vi "MainController4.vi"() -> ()   [LabVIEW 2009]
doc: "The top-level VI for the SRV application.\n\n\nModified: Mike Schultz - Logic PD"
uses:
  SRV VIs/ImageProcessing/QT_Image.ctl
  SRV VIs/SubVIs/SRV_Response Data Type.ctl
  SRV VIs/Motors/Motors Config/SRV_Motor Control Button Icons_TRUE.ctl
  SRV VIs/Motors/Motors Config/SRV_Motor Control Button Icons_FALSE.ctl
  SRV VIs/SubVIs/SRV_SRV_Loops Notifier Methods.ctl
  SRV VIs/SRV_Main Controller Local Data.ctl
  SRV VIs/Motors/Motors Config/SRV_Motor Control Button Config.ctl
  SRV VIs/Motors/Motors Config/SRV_Motor Legos-Servo.ctl
  SRV VIs/Motors/Motors Config/SRV_Motor Control Commands Cluster.ctl
  SRV VIs/Motors/Motors Config/SRV_Motor Control Command Config.ctl
  SRV VIs/SubVIs/SRV_Streaming States.ctl
  SRV VIs/SubVIs/SRV_Streaming State.ctl
  SRV VIs/PacketMode/SRV_PM_Packet.ctl
  SRV VIs/Support/SRV_Command-Data Queue Data Type.ctl
  SRV VIs/PacketMode/SRV_PM_Packet Mode Style.ctl
  SRV VIs/Motors/SRV_Button Event Data.ctl
  SRV VIs/SubVIs/SRV_Streaming Modes.ctl
  <vilib>/Utility/miscctls.llb/LVBoundsTypeDef.ctl
  SRV VIs/SubVIs/SRV_Number of IMJ Requests Methods.ctl
  SRV VIs/SubVIs/SRVGlobals.vi
panel:
  in  "button E5":bool
  out "true E5":T1
  out "false E5":T2
  in  "button E4":bool
  out "true E4":T1
  out "false E4":T2
  in  "button E3":bool
  out "true E3":T1
  out "false E3":T2
  in  "button E1":bool
  out "true E1":T1
  out "false E1":T2
  in  "button E2":bool
  out "true E2":T1
  out "false E2":T2
  in  "button E7":bool
  out "true E7":T1
  out "false E7":T2
  in  "button E6":bool
  out "true E6":T1
  out "false E6":T2
  in  "button D7":bool
  out "true D7":T1
  out "false D7":T2
  in  "button A7":bool
  out "true A7":T1
  out "false A7":T2
  in  "button C7":bool
  out "true C7":T1
  out "false C7":T2
  in  "button B7":bool
  out "true B7":T1
  out "false B7":T2
  in  "button D6":bool
  out "true D6":T1
  out "false D6":T2
  in  "button A6":bool
  out "true A6":T1
  out "false A6":T2
  in  "button C6":bool
  out "true C6":T1
  out "false C6":T2
  in  "button B6":bool
  out "true B6":T1
  out "false B6":T2
  in  "button D5":bool
  out "true D5":T1
  out "false D5":T2
  in  "button A5":bool
  out "true A5":T1
  out "false A5":T2
  in  "button C5":bool
  out "true C5":T1
  out "false C5":T2
  in  "button B5":bool
  out "true B5":T1
  out "false B5":T2
  in  "button D4":bool
  out "true D4":T1
  out "false D4":T2
  in  "button A4":bool
  out "true A4":T1
  out "false A4":T2
  in  "button C4":bool
  out "true C4":T1
  out "false C4":T2
  in  "button B4":bool
  out "true B4":T1
  out "false B4":T2
  in  "button D3":bool
  out "true D3":T1
  out "false D3":T2
  in  "button A3":bool
  out "true A3":T1
  out "false A3":T2
  in  "button C3":bool
  out "true C3":T1
  out "false C3":T2
  in  "button B3":bool
  out "true B3":T1
  out "false B3":T2
  in  "button D2":bool
  out "true D2":T1
  out "false D2":T2
  in  "button A2":bool
  out "true A2":T1
  out "false A2":T2
  in  "button C2":bool
  out "true C2":T1
  out "false C2":T2
  in  "button B2":bool
  out "true B2":T1
  out "false B2":T2
  in  "Expand-Collapse":bool
  in  "button D1":bool
  out "true D1":T1
  out "false D1":T2
  in  "button A1":bool
  out "true A1":T1
  out "false A1":T2
  in  "button C1":bool
  out "true C1":T1
  out "false C1":T2
  in  "button B1":bool
  out "true B1":T1
  out "false B1":T2
  out "Overflow Indicator":bool
  out "ms Diff 3":u32
  out "ms Diff 2":u32
  out "ms Diff parse":u32
  out "ms Diff ##IMJ":u32
  out "ms Diff DQ":u32
  out "ms Diff":u32
  out "Response Data Type":T3=enum."No Data"
  out "i4":i32
  in  "Show Image":bool
  out "InPico State Change":bool
  in  "clear":bool
  out "Replies":string
  out "Number of IMJ Requests":i32
  out "XModem Replies":string[](array[string])
  out "i1":i32
  out "i2":i32
  out "Status":string
  out "The image":picture caption="new picture"
  out "SRV Out":refnum<k5>
  out "SRV IP Address":string
  out "In Pico":bool
  out "connected?":bool
  in  "Tab Control":T4(tab)
  in  "Send Text":bool
  in  "ESC":bool
  in  "Direct Command to Send":string
  in  "Run CCode":bool
  in  "View Code":bool
  in  "Upload CCode":bool
  in  "C Code":string="int x,y,z;\nfor (x = 0; x < 2; x++) \n  {  \n    for (y = 0; y < 3; y++)\n       {       \n         for (z = 0; z < 2; z++)\n           {\n             printf(\"%d %d %d\\n\", x,y,z);   \n           }\n        } \n   }\nexit(1);"
  in  "load Text":bool
  out "Cover":bool
  out "Last file name":string
  in  "Movie Mode":bool
  in  "Path to folder":path
  in  "Snap":bool
  out "YUV_SRV":cluster{"Y":sgl, "U":sgl, "V":sgl}
  in  "Threshold":i8(slide)=4 scale=1.0..9.0
  in  "Plan":T5(radio)
  in  "Bins":T6(ring)=enum."4 levels of U and 4 levels of V"
  out "Image/Movie Out":T7 {"Dialogs" format="%.0b"}
  out "YUV_Calc":cluster{"Y":sgl, "U":sgl, "V":sgl}
  in  "firmware":path
  in  "Upload":bool
  in  "Version":bool
  in  "Edit Sensors Config":bool
  in  "Edit System Config":bool
  out "System Config":string
  in  "Edit Motors Config":bool
  in  "stop":bool
  # "SRV Communication"
  # "Debug indicators below.\nA developer just needs to enlarge the decoration to include these at debug time."
  # "To use movie feature, turn Movie Mode on and then hit Snap to start recording. Turn Movie Mode off to stop recording."
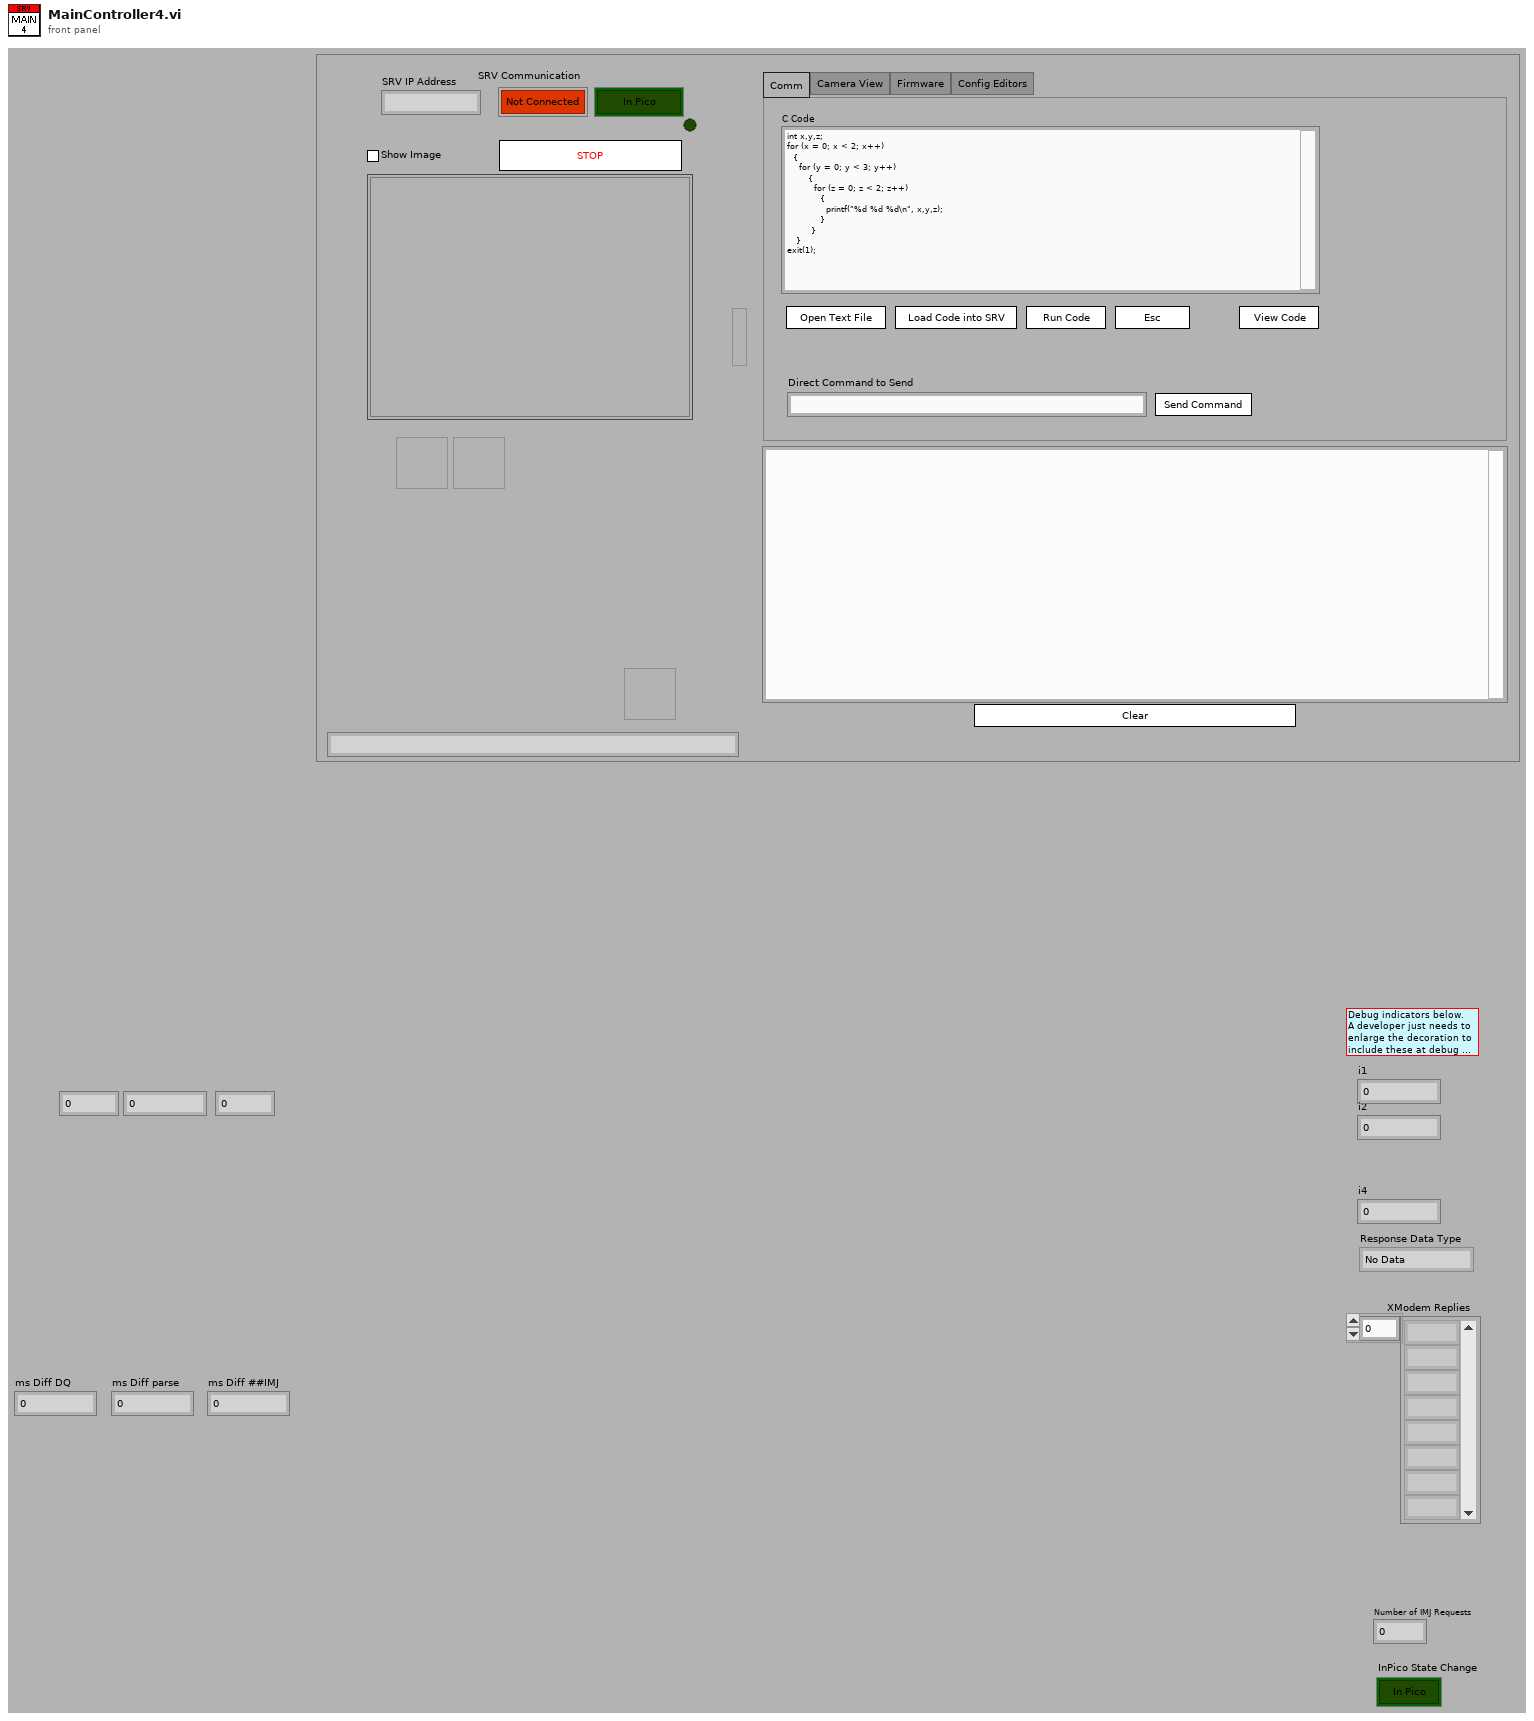
[diagram p1: front panel]
types:
  T1 = typedef "SRV_Motor Control Button Icons_TRUE.ctl" = u16
  T2 = typedef "SRV_Motor Control Button Icons_FALSE.ctl" = u16
  T3 = typedef "SRV_Response Data Type.ctl" = enum16{"Undefined Data", "##IMJ", "#B", "Leaving PicoC", "##vp", "##zZ", "#NA", "##$A", "#NB", "##il", "##iL", "##NP,", "##R,", "No Data"}
  T4 = enum32{"Comm", "Camera View", "Firmware", "Config Editors"}
  T5 = enum32{"Nothing", "Differencing", "Color Segmentation", "Edge detection", "Horizon detection", "Obstacle detection"}
  T6 = enum16{"Zero all", "4 levels of Y, 2 levels of U, 2 levels of V", "4 levels of U and 4 levels of V", "even distribution across U and V", "16 grayscale levels"}
  T7 = typedef "QT_Image.ctl" = cluster{"Witdh":i32, "Height":i32, "Depth":i32, "data":u8[], "Compressed data":u8[], "Color table":u32[], "Duration":i32, "Options":i32, "Timestamp":i32, "ID":i32, "Reserved":i32, "Dialogs":u32}
  T8 = typedef "SRV_Main Controller Local Data.ctl" = cluster{"user event":refnum<user-event>, "SRV":refnum<k5>, "Replies":refnum<vi>, "Status":refnum<vi>, "false refs":refnum<vi>[], "true refs":refnum<vi>[], "Motor Control Config":T9[], "Default Config Dir":path, "System Config Name":string, "Cached Streaming States":T13, "Main Controller ref":refnum<vi>, "Sensor View ref":refnum<vi>, "VISTA or Later?":bool, "button refs":refnum<vi>[]}
  T9 = typedef "SRV_Motor Control Button Config.ctl" = cluster{"Button Name":string, "Button Label":string, "Motor Type":T10, "Press Cmds":T11, "Release Cmds":T11, "Icon":T2}
  T10 = typedef "SRV_Motor Legos-Servo.ctl" = enum16{"Servo", "Legos", "Shared Var"}
  T11 = typedef "SRV_Motor Control Commands Cluster.ctl" = cluster{"Motor Control Commands Array":T12[]}
  T12 = typedef "SRV_Motor Control Command Config.ctl" = cluster{"I2C Address":u8, "Register":u8, "Value":u8, "Active":bool}
  T13 = typedef "SRV_Streaming States.ctl" = cluster{"Video":T14, "Sensors":T14}
  T14 = typedef "SRV_Streaming State.ctl" = cluster{"Enabled":bool, "Data":string}
  T15 = typedef "SRV_SRV_Loops Notifier Methods.ctl" = enum16{"Wait on Notification", "Send Notification", "Release Notifier"}
  T16 = typedef "SRV_PM_Packet.ctl" = cluster{"Packet Data":u8[], "Header Complete?":bool, "Complete?":bool, "Checksum OK?":bool, "Error?":bool}
  T17 = enum8{"Enabled", "Disabled", "Disabled and Grayed Out"}
  T18 = typedef "SRV_Command-Data Queue Data Type.ctl" = cluster{"Command":string, "Data":variant}
  T19 = typedef "SRV_PM_Packet Mode Style.ctl" = enum16{"Old", "New PM"}
  T20 = typedef "Semaphore RefNum" = refnum<k1>
  T21 = typedef "SRV_Button Event Data.ctl" = cluster{"Button NewVal":bool, "Button Index":i32}
  T22 = enum16{"Disable", "Frame Differencing", "Color Segmentation", "Edge Detection", "Horizon detection", "Obstacle detection", "Stereo processing"}
  T23 = typedef "SRV_Streaming Modes.ctl" = enum16{"Video", "Sensors"}
  T24 = typedef "LVBoundsTypeDef.ctl" = cluster{"Width":u32, "Height":u32}
  T25 = typedef "SRV_Number of IMJ Requests Methods.ctl" = enum16{"Read", "Increment", "Decrement", "Reset", "Close"}
  T26 = typedef "SRV_System Config.ctl" = cluster{"SRV IP Address":string, "Video Stream Rate Period (ms)":u32, "Enable Diagnostic Log":bool, "Watchdog 1 Config":T27, "Watchdog 2 Config":T27, "Sensor Window Filepath":path}
  T27 = typedef "SRV_Watchdog Config Cluster.ctl" = cluster{"Watchdog Name":string, "Watchdog Period (s)":dbl, "Watchdog Command":T12}
  T28 = typedef "LVMouseTypeDef.ctl" = cluster{"Mouse Position":cluster{"X":i32, "Y":i32}, "Mouse Modifiers":cluster{"Button Down":bool, "Shift Mod":bool, "Menu Mod":bool, "Option Mod":bool}}
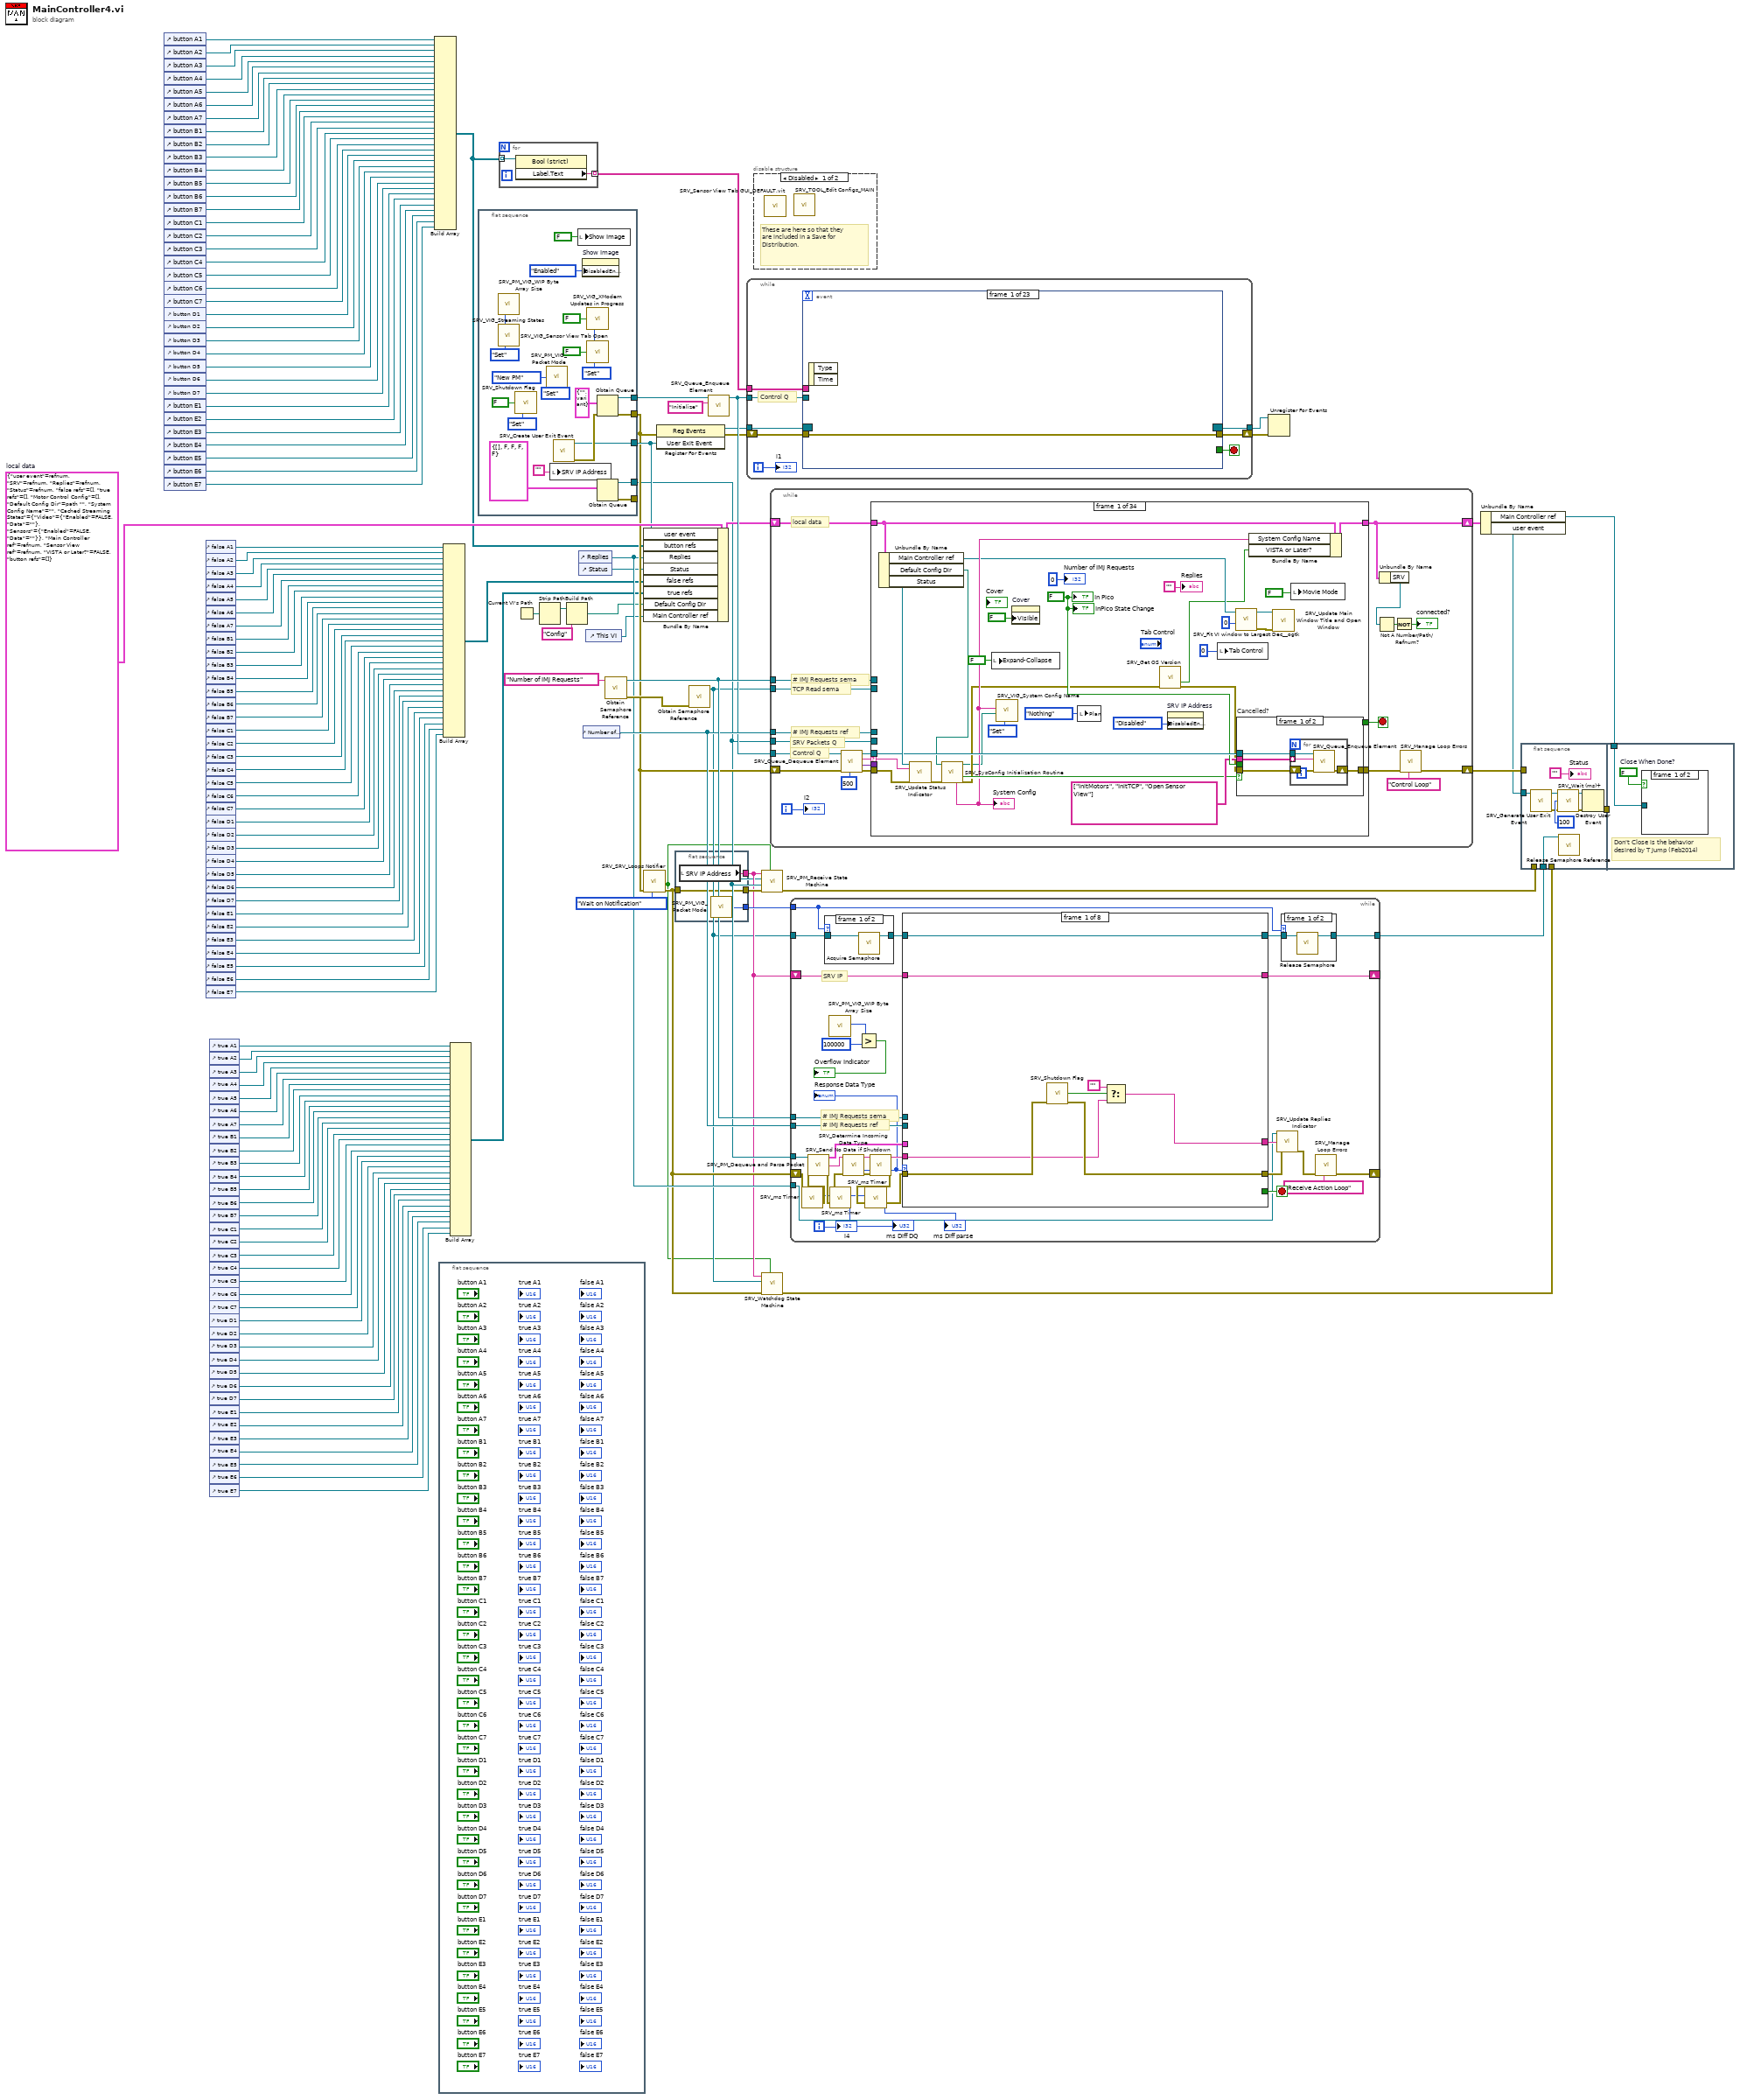
[diagram p0: block diagram]
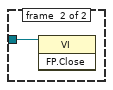
[diagram p3: hidden frame]
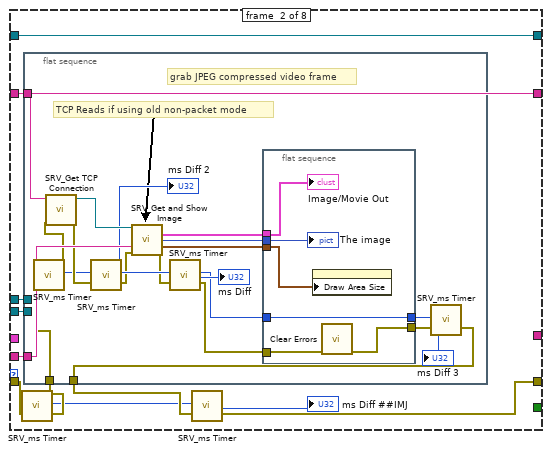
[diagram p6: hidden frame]
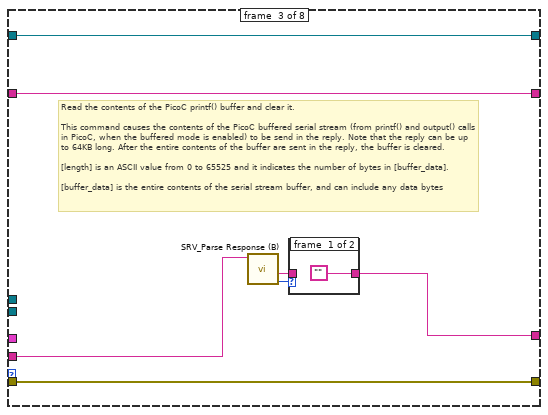
[diagram p7: hidden frame]
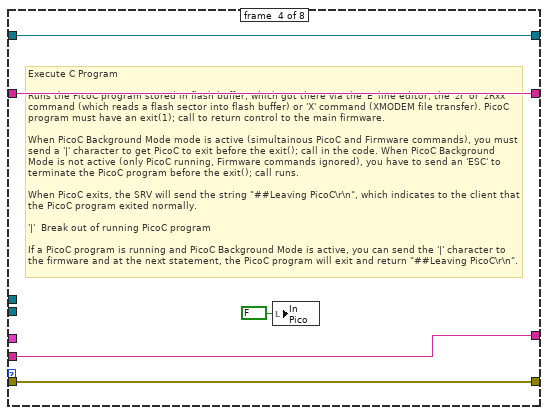
[diagram p9: hidden frame]
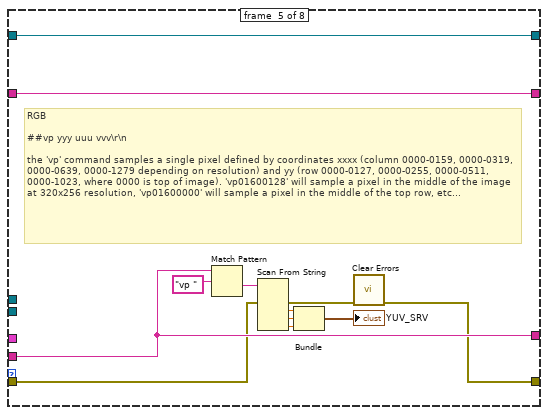
[diagram p10: hidden frame]
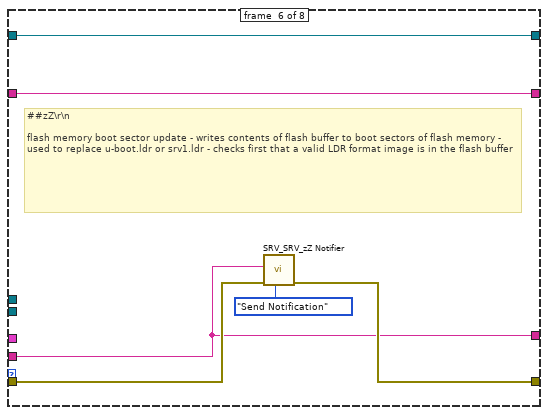
[diagram p11: hidden frame]
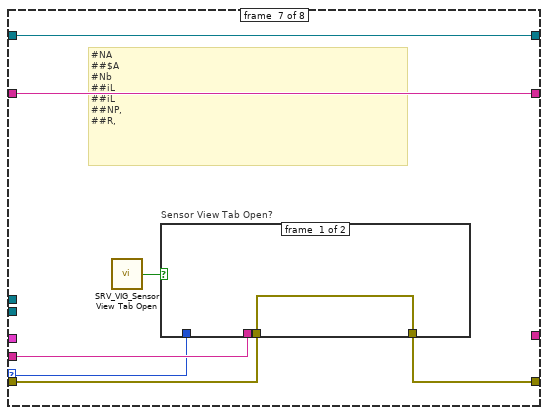
[diagram p12: hidden frame]
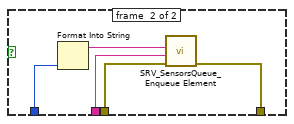
[diagram p13: hidden frame]
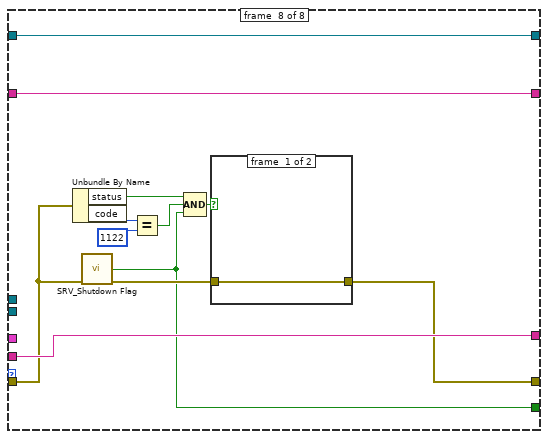
[diagram p14: hidden frame]
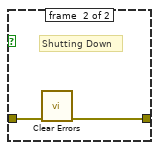
[diagram p15: hidden frame]
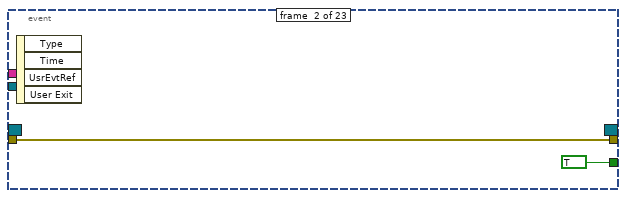
[diagram p16: hidden frame]
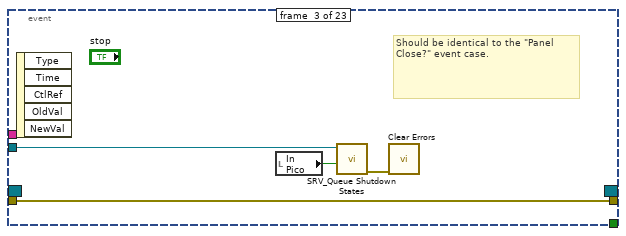
[diagram p17: hidden frame]
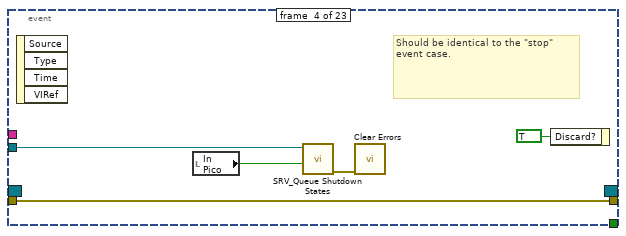
[diagram p18: hidden frame]
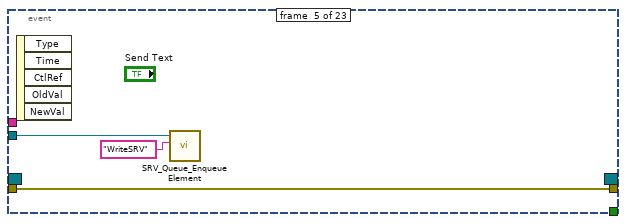
[diagram p19: hidden frame]
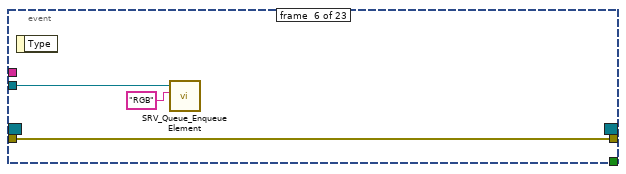
[diagram p20: hidden frame]
diagram:
  w136 = T8 {"user event"=refnum, "SRV"=refnum, "Replies"=refnum, "Status"=refnum, "false refs"=[], "true refs"=[], "Motor Control Config"=[], "Default Config Dir"=path "", "System Config Name"="", "Cached Streaming States"={"Video"={"Enabled"=FALSE, "Data"=""}, "Sensors"={"Enabled"=FALSE, "Data"=""}}, "Main Controller ref"=refnum, "Sensor View ref"=refnum, "VISTA or Later?"=FALSE, "button refs"=[]}  # local data
  n1 = control-ref of="button A1"() -> (w106:refnum<vi>)
  n2 = control-ref of="button A2"() -> (w105:refnum<vi>)
  n3 = control-ref of="button A3"() -> (w104:refnum<vi>)
  n4 = control-ref of="button A4"() -> (w103:refnum<vi>)
  n5 = control-ref of="button A5"() -> (w102:refnum<vi>)
  n6 = control-ref of="button A6"() -> (w101:refnum<vi>)
  n7 = control-ref of="button A7"() -> (w100:refnum<vi>)
  n8 = control-ref of="button B1"() -> (w99:refnum<vi>)
  n9 = control-ref of="button B2"() -> (w98:refnum<vi>)
  n10 = control-ref of="button B3"() -> (w97:refnum<vi>)
  n11 = control-ref of="button B4"() -> (w96:refnum<vi>)
  n12 = control-ref of="button B5"() -> (w95:refnum<vi>)
  n13 = control-ref of="button B6"() -> (w94:refnum<vi>)
  n14 = control-ref of="button B7"() -> (w93:refnum<vi>)
  n15 = control-ref of="button C1"() -> (w92:refnum<vi>)
  n16 = control-ref of="button C2"() -> (w91:refnum<vi>)
  n17 = control-ref of="button C3"() -> (w90:refnum<vi>)
  n18 = control-ref of="button C4"() -> (w89:refnum<vi>)
  n19 = control-ref of="button C5"() -> (w88:refnum<vi>)
  n20 = control-ref of="button C6"() -> (w87:refnum<vi>)
  n21 = control-ref of="button C7"() -> (w86:refnum<vi>)
  n22 = control-ref of="button D1"() -> (w85:refnum<vi>)
  n23 = control-ref of="button D2"() -> (w84:refnum<vi>)
  n24 = control-ref of="button D3"() -> (w83:refnum<vi>)
  n25 = control-ref of="button D4"() -> (w82:refnum<vi>)
  n26 = control-ref of="button D5"() -> (w81:refnum<vi>)
  n27 = control-ref of="button D6"() -> (w80:refnum<vi>)
  n28 = control-ref of="button D7"() -> (w79:refnum<vi>)
  n29 = control-ref of="button E1"() -> (w21:refnum<vi>)
  n30 = control-ref of="button E2"() -> (w20:refnum<vi>)
  n31 = control-ref of="button E3"() -> (w19:refnum<vi>)
  n32 = control-ref of="button E4"() -> (w18:refnum<vi>)
  n33 = control-ref of="button E5"() -> (w17:refnum<vi>)
  n34 = control-ref of="button E6"() -> (w16:refnum<vi>)
  n35 = control-ref of="button E7"() -> (w15:refnum<vi>)
  n36 = control-ref of="false A1"() -> (w50:refnum<vi>)
  n37 = control-ref of="false A2"() -> (w49:refnum<vi>)
  n38 = control-ref of="false A3"() -> (w48:refnum<vi>)
  n39 = control-ref of="false A4"() -> (w47:refnum<vi>)
  n40 = control-ref of="false A5"() -> (w46:refnum<vi>)
  n41 = control-ref of="false A6"() -> (w45:refnum<vi>)
  n42 = control-ref of="false A7"() -> (w44:refnum<vi>)
  n43 = control-ref of="false B1"() -> (w43:refnum<vi>)
  n44 = control-ref of="false B2"() -> (w42:refnum<vi>)
  n45 = control-ref of="false B3"() -> (w41:refnum<vi>)
  n46 = control-ref of="false B4"() -> (w40:refnum<vi>)
  n47 = control-ref of="false B5"() -> (w39:refnum<vi>)
  n48 = control-ref of="false B6"() -> (w38:refnum<vi>)
  n49 = control-ref of="false B7"() -> (w37:refnum<vi>)
  n50 = control-ref of="false C1"() -> (w36:refnum<vi>)
  n51 = control-ref of="false C2"() -> (w35:refnum<vi>)
  n52 = control-ref of="false C3"() -> (w34:refnum<vi>)
  n53 = control-ref of="false C4"() -> (w33:refnum<vi>)
  n54 = control-ref of="false C5"() -> (w32:refnum<vi>)
  n55 = control-ref of="false C6"() -> (w31:refnum<vi>)
  n56 = control-ref of="false C7"() -> (w30:refnum<vi>)
  n57 = control-ref of="false D1"() -> (w29:refnum<vi>)
  n58 = control-ref of="false D2"() -> (w28:refnum<vi>)
  n59 = control-ref of="false D3"() -> (w27:refnum<vi>)
  n60 = control-ref of="false D4"() -> (w26:refnum<vi>)
  n61 = control-ref of="false D5"() -> (w25:refnum<vi>)
  n62 = control-ref of="false D6"() -> (w24:refnum<vi>)
  n63 = control-ref of="false D7"() -> (w23:refnum<vi>)
  n64 = control-ref of="false E1"() -> (w7:refnum<vi>)
  n65 = control-ref of="false E2"() -> (w6:refnum<vi>)
  n66 = control-ref of="false E3"() -> (w5:refnum<vi>)
  n67 = control-ref of="false E4"() -> (w4:refnum<vi>)
  n68 = control-ref of="false E5"() -> (w3:refnum<vi>)
  n69 = control-ref of="false E6"() -> (w2:refnum<vi>)
  n70 = control-ref of="false E7"() -> (w1:refnum<vi>)
  n71 = control-ref of="true A1"() -> (w78:refnum<vi>)
  n72 = control-ref of="true A2"() -> (w77:refnum<vi>)
  n73 = control-ref of="true A3"() -> (w76:refnum<vi>)
  n74 = control-ref of="true A4"() -> (w75:refnum<vi>)
  n75 = control-ref of="true A5"() -> (w74:refnum<vi>)
  n76 = control-ref of="true A6"() -> (w73:refnum<vi>)
  n77 = control-ref of="true A7"() -> (w72:refnum<vi>)
  n78 = control-ref of="true B1"() -> (w71:refnum<vi>)
  n79 = control-ref of="true B2"() -> (w70:refnum<vi>)
  n80 = control-ref of="true B3"() -> (w69:refnum<vi>)
  n81 = control-ref of="true B4"() -> (w68:refnum<vi>)
  n82 = control-ref of="true B5"() -> (w67:refnum<vi>)
  n83 = control-ref of="true B6"() -> (w66:refnum<vi>)
  n84 = control-ref of="true B7"() -> (w65:refnum<vi>)
  n85 = control-ref of="true C1"() -> (w64:refnum<vi>)
  n86 = control-ref of="true C2"() -> (w63:refnum<vi>)
  n87 = control-ref of="true C3"() -> (w62:refnum<vi>)
  n88 = control-ref of="true C4"() -> (w61:refnum<vi>)
  n89 = control-ref of="true C5"() -> (w60:refnum<vi>)
  n90 = control-ref of="true C6"() -> (w59:refnum<vi>)
  n91 = control-ref of="true C7"() -> (w58:refnum<vi>)
  n92 = control-ref of="true D1"() -> (w57:refnum<vi>)
  n93 = control-ref of="true D2"() -> (w56:refnum<vi>)
  n94 = control-ref of="true D3"() -> (w55:refnum<vi>)
  n95 = control-ref of="true D4"() -> (w54:refnum<vi>)
  n96 = control-ref of="true D5"() -> (w53:refnum<vi>)
  n97 = control-ref of="true D6"() -> (w52:refnum<vi>)
  n98 = control-ref of="true D7"() -> (w51:refnum<vi>)
  n99 = control-ref of="true E1"() -> (w14:refnum<vi>)
  n100 = control-ref of="true E2"() -> (w13:refnum<vi>)
  n101 = control-ref of="true E3"() -> (w12:refnum<vi>)
  n102 = control-ref of="true E4"() -> (w11:refnum<vi>)
  n103 = control-ref of="true E5"() -> (w10:refnum<vi>)
  n104 = control-ref of="true E6"() -> (w9:refnum<vi>)
  n105 = control-ref of="true E7"() -> (w8:refnum<vi>)
  n106 = Build Array(w106, w105, w104, w103, w102, w101, w100, w99, w98, w97, w96, w95, w94, w93, w92, w91, w90, w89, w88, w87, w86, w85, w84, w83, w82, w81, w80, w79, w21, w20, w19, w18, w17, w16, w15) -> (w22:refnum<vi>[])
  n107 = flat-sequence {
    frame #0 {
    }
  }
  n108 = Build Array(w50, w49, w48, w47, w46, w45, w44, w43, w42, w41, w40, w39, w38, w37, w36, w35, w34, w33, w32, w31, w30, w29, w28, w27, w26, w25, w24, w23, w7, w6, w5, w4, w3, w2, w1) -> (w122:refnum<vi>[])
  n109 = Build Array(w78, w77, w76, w75, w74, w73, w72, w71, w70, w69, w68, w67, w66, w65, w64, w63, w62, w61, w60, w59, w58, w57, w56, w55, w54, w53, w52, w51, w14, w13, w12, w11, w10, w9, w8) -> (w121:refnum<vi>[])
  n110 = flat-sequence {
    tunnel: [w160] -> w137
    tunnel: [w161] -> w132
    tunnel: [w158] -> w133
    tunnel: [w153] -> w114
    tunnel: [w152] -> _
    frame #0 {
      w149 = enum16{"Get", "Set"}."Set" ("Method (Get)")
      w150 = enum16{"Get", "Set"}."Set" ("Method (Get)")
      n111 = call "SRV_PM_VIG_WIP Byte Array Size.vi"("Method (Get)"=w150) -> ()  [unwired: 9 in, 2 out]
      n112 = call "SRV_VIG_Streaming States.vi"("Method (Get)"=w150) -> ()  [unwired: 14 in, 1 out]
      n113 = call "SRV_Shutdown Flag.vi"("Shutdown Flag"=FALSE, "Method (Get)"=enum16{"Get", "Set"}."Set") -> ()  [unwired: 12 in, 2 out]
      n114 = call "SRV_PM_VIG_Packet Mode.vi"("Packet Mode Style"=SRV_PM_Packet_Mode_Style."New PM", "Method (Get)"=enum16{"Get", "Set"}."Set") -> ()  [unwired: 13 in, 1 out]
      n115 = local write "SRV IP Address"("") -> ()
      n116 = call "SRV_Create User Exit Event.vi"() -> ("error out"=w159:errorcluster, "User Exit Event"=w158:refnum<user-event>)  [unwired: 10 in]
      n117 = local write "Show Image"(FALSE ("Show Image")) -> ()
      n118 = property on="Show Image" class="Bool (strict)"("DisabledEnum"=T17."Enabled" ("Disabled")) -> ()  [unwired: 2 in, 2 out]
      n119 = call "SRV_VIG_XModem Updates in Progress.vi"("XModem Updates in Progress"=FALSE, "Method (Get)"=w149) -> ()  [unwired: 12 in, 2 out]
      n120 = call "SRV_VIG_Sensor View Tab Open.vi"("Sensor View Tab Open"=FALSE, "Method (Get)"=w149) -> ()  [unwired: 12 in, 2 out]
      n121 = Obtain Queue(element data type=T18 {"Command"="", "Data"=variant} ("Queue Data Type"), error in (no error)=w159) -> (queue out=w160:refnum<queue>, error out=w161:errorcluster)  [unwired: 3 in, 1 out]
      n122 = Obtain Queue(element data type=T16 {"Packet Data"=[], "Header Complete?"=FALSE, "Complete?"=FALSE, "Checksum OK?"=FALSE, "Error?"=FALSE} ("Packet")) -> (queue out=w153:refnum<queue>, error out=w152:errorcluster)  [unwired: 4 in, 1 out]
    }
  }
  n123 = for {
    tunnel: w22 -> [w168] mode=indexing
    tunnel: [w167] -> w120 mode=indexing
    n124 = property class="Bool (strict)"(reference=w168) -> ("Label.Text"=w167:string)  [unwired: 1 in, 2 out]
  }
  n125 = Current VI's Path() -> (path=w118:path)
  n126 = Strip Path(path=w118) -> (stripped path=w119:path)  [unwired: 1 out]
  n127 = Build Path(base path=w119, name or relative path="Config") -> (appended path=w116:path)
  n128 = control-ref of="Replies"() -> (w124:refnum<vi>)
  n129 = control-ref of="Status"() -> (w123:refnum<vi>)
  n130 = control-ref of="Number of IMJ Requests"() -> (w141:refnum<vi>)
  n131 = control-ref of="This VI"() -> (w113:refnum<vi>)
  n132 = call <vilib>:"Obtain Semaphore Reference.vi"("name (unnamed)"="Number of IMJ Requests") -> ("error out"=w145:errorcluster, "semaphore"=w142:T20)  [unwired: 4 in, 1 out]
  n133 = Bundle By Name(cluster=w136, "user event"=w133, "button refs"=w22, "Replies"=w124, "Status"=w123, "false refs"=w122, "true refs"=w121, "Default Config Dir"=w116, "Main Controller ref"=w113) -> (w135:T8)
  n134 = call "SRV_SRV_Loops Notifier.vi"("Notifier Methods"=SRV_SRV_Loops_Notifier_Methods."Wait on Notification", "error in (no error)"=w132) -> ("error out"=w111:errorcluster, "Cancelled?"=w108:bool)  [unwired: 8 in]
  n135 = register-events(error in=w132, w133) -> (reference out=w131:refnum<event-registration>, error out=w134:errorcluster)  [unwired: 1 in]
  n136 = flat-sequence {
    tunnel: [w171] -> w143
    tunnel: w111 -> [w171]
    tunnel: [w170] -> w110
    tunnel: [w169] -> w139
    frame #0 {
      n137 = local read "SRV IP Address"() -> (w170:string)
      n138 = call "SRV_PM_VIG_Packet Mode.vi"() -> ("Packet Mode Style"=w169:T19)  [unwired: 15 in]
    }
  }
  n139 = call <vilib>:"Obtain Semaphore Reference.vi"("error in (no error)"=w145) -> ("semaphore"=w109:T20)  [unwired: 4 in, 2 out]
  n140 = call "SRV_Queue_Enqueue Element.vi"("Command"="Initialize" ("name (unnamed)"), "Command-Data Queue"=w137) -> ("Command-Data Queue out"=w138:refnum<queue>)  [unwired: 7 in, 2 out]
  n141 = while {
    tunnel: w138 -> [w179]
    shift-right: [w174] -> w130
    shift-left: w134 -> [w175]
    tunnel: w131 -> [w176]
    tunnel: [w173] -> w129
    tunnel: w120 -> [w172]
    i -> [w177]
    stop <- w178 stop-if-true
    # "Control Q"
    n142 = event shown="[22] \"button A1\", \"button A2\", \"button A3\", \"button A4\", \"button A5\", \"button A6\", \"button A7\", \"button B1\", \"button B2\", \"button B3\", \"button B4\", \"button B5\", \"button B6\", \"button B7\", \"button C1\", \"button C2\", \"button C3\", \"button C4\", \"button C5\", \"button C6\", \"button C7\", \"button D1\", \"button D2\", \"button D3\", \"button D4\", \"button D5\", \"button D6\", \"button D7\", \"button E1\", \"button E2\", \"button E3\", \"button E4\", \"button E5\", \"button E6\", \"button E7\": Value Change" {
      selector: w176 -> [_ _ _ _ _ _ _ _ _ _ _ _ _ _ _ _ _ _ _ _ _ _ _]
      dyn-events: [_ _ _ _ _ _ _ _ _ _ _ _ _ _ _ _ _ _ _ _ _ _ _] -> w173
      timeout: _ -> [_ _ _ _ _ _ _ _ _ _ _ _ _ _ _ _ _ _ _ _ _ _ _]
      tunnel: w179 -> [_ _ w185 w189 w193 w196 w199 _ w214 w246 w257 w268 w279 w290 w301 w308 w311 w314 w320 w324 w328 w332 w344]
      tunnel: [_ TRUE ("stop") _ _ _ _ _ _ _ _ _ _ _ _ _ _ _ _ _ _ _ _ _] -> w178
      tunnel: w175 -> [w180 w181 w183 w187 w192 w195 w198 w201 w213 w244 w252 w263 w274 w285 w296 w307 w310 w313 w318 w322 w326 w330 w341]
      tunnel: [w180 w181 w183 w187 w192 w195 w198 w201 w213 w244 w252 w263 w274 w285 w296 w307 w310 w313 w317 w321 w325 w329 w343] -> w174
      tunnel: w172 -> [_ _ _ _ _ _ _ _ _ _ _ _ _ _ _ _ _ _ _ _ _ _ w339]
      event #0 {
        n143 = event-data() -> ()  [unwired: 1 in, 2 out]
      }
      event #1 {
        n144 = event-data() -> ()  [unwired: 1 in, 4 out]
      }
      event #2 {
        # "Should be identical to the \"Panel Close?\" event case."
        n145 = event-data() -> ()  [unwired: 1 in, 5 out]
        n146 = local read "In Pico"() -> (w186:bool)
        n147 = call "SRV_Queue Shutdown States.vi"("In Pico"=w186, "Control Queue"=w185) -> ("error out"=w184:errorcluster)  [unwired: 8 in, 1 out]
        n148 = call <vilib>:"Clear Errors.vi"("error in (no error)"=w184) -> ()  [unwired: 6 in, 1 out]
      }
      event #3 {
        # "Should be identical to the \"stop\" event case."
        n149 = event-data() -> ()  [unwired: 1 in, 4 out]
        n150 = local read "In Pico"() -> (w188:bool)
        n151 = call "SRV_Queue Shutdown States.vi"("In Pico"=w188, "Control Queue"=w189) -> ("error out"=w190:errorcluster)  [unwired: 8 in, 1 out]
        n152 = call <vilib>:"Clear Errors.vi"("error in (no error)"=w190) -> ()  [unwired: 6 in, 1 out]
        n153 = event-data("Discard?"=TRUE) -> ()  [unwired: 1 in, 1 out]
      }
      event #4 {
        n154 = event-data() -> ()  [unwired: 1 in, 5 out]
        n155 = call "SRV_Queue_Enqueue Element.vi"("Command"="WriteSRV" ("name (unnamed)"), "Command-Data Queue"=w193) -> ()  [unwired: 7 in, 3 out]
      }
      event #5 {
        n156 = event-data() -> ()  [unwired: 1 in, 1 out]
        n157 = call "SRV_Queue_Enqueue Element.vi"("Command"="RGB" ("name (unnamed)"), "Command-Data Queue"=w196) -> ()  [unwired: 7 in, 3 out]
      }
      event #6 {
        n158 = event-data() -> ()  [unwired: 1 in, 1 out]
        n159 = call "SRV_Queue_Enqueue Element.vi"("Command"="Snap" ("name (unnamed)"), "Command-Data Queue"=w199) -> ()  [unwired: 7 in, 3 out]
      }
      event #7 {
        n160 = event-data() -> ()  [unwired: 1 in, 1 out]
        n161 = call "File Dialog2"("prompt"="Select a C code text file...", "pattern (all files)"="*.c;*.txt", "pattern label"="C Code Text File") -> ("selected path"=w202:path, "error out"=w203:errorcluster)  [unwired: 9 in, 2 out]
        n162 = case shown="No Error" w203 {
          selector: w203 -> [w208 _]
          tunnel: w202 -> [w207 _]
          frame #0 {
            n163 = Read from Text File(file (use dialog)=w207, error in=w208) -> (text=w209:string, error out=w210:errorcluster)  [unwired: 2 in, 2 out]
            n164 = case shown="No Error" w210 {
              tunnel: w209 -> [w211 _]
              frame #0 {
                n165 = local write "C Code"(w211) -> ()
              }
              frame #1 {
              }
            }
          }
          frame #1 {
          }
        }
      }
      event #8 {
        n166 = event-data() -> ()  [unwired: 1 in, 1 out]
        n167 = local read "firmware"() -> (w215:path)
        n168 = Empty String/Path?(string/path=w215) -> (empty?=w218:bool)
        n169 = case shown="True" w218 {
          tunnel: [FALSE ("cancelled") w236] -> w217
          tunnel: [w233 w235] -> w216
          tunnel: w215 -> [w233 _]
          frame #0 {
          }
          frame #1 {
            n170 = call "File Dialog3"("prompt"="Select a firmware file...", "pattern (all files)"="*.ldr", "pattern label"="Firmware File") -> ("selected path"=w235:path, "cancelled"=w236:bool, "error out"=w234:errorcluster)  [unwired: 9 in, 1 out]
            n171 = call <vilib>:"Clear Errors.vi"("error in (no error)"=w234) -> ()  [unwired: 6 in, 1 out]
          }
        }
        n172 = property on="Show Image" class="Bool (strict)"("DisabledEnum"=T17."Disabled and Grayed Out" ("Disabled")) -> ()  [unwired: 2 in, 2 out]
        n173 = case shown="False" w217 {
          tunnel: w214 -> [w224 _]
          tunnel: w216 -> [w222 _]
          frame #0 {
            n174 = flat-sequence {
              tunnel: [w225] -> w223
              tunnel: w222 -> [w226]
              frame #0 {
                n175 = local write "firmware"(w226) -> ()
                n176 = local read "In Pico"() -> (w225:bool)
              }
            }
            n177 = case shown="True" w223 {
              tunnel: w224 -> [w227 w230]
              tunnel: [w227 w229] -> w220
              tunnel: [_ w228] -> w219
              frame #0 {
              }
              frame #1 {
                n178 = call "SRV_Queue_Enqueue Element.vi"("Command"="Escape" ("name (unnamed)"), "Command-Data Queue"=w230) -> ("error out"=w228:errorcluster, "Command-Data Queue out"=w229:refnum<queue>)  [unwired: 7 in, 1 out]
              }
            }
            n179 = call "SRV_Queue Streaming Halt and Restore States.vi"("error in (no error)"=w219, "Commands"=T18[] [{"Command"="Upload", "Data"=variant}, {"Command"="Boot", "Data"=variant}], "Control Queue"=w220) -> ()  [unwired: 7 in, 2 out]
          }
          frame #1 {
          }
        }
      }
      event #9 {
        n180 = event-data() -> ()  [unwired: 1 in, 1 out]
        n181 = local read "In Pico"() -> (w245:bool)
        n182 = case shown="True" w245 {
          tunnel: w246 -> [w247 w250]
          tunnel: [w247 w249] -> w243
          tunnel: [_ w248] -> w242
          frame #0 {
          }
          frame #1 {
            n183 = call "SRV_Queue_Enqueue Element.vi"("Command"="Escape" ("name (unnamed)"), "Command-Data Queue"=w250) -> ("error out"=w248:errorcluster, "Command-Data Queue out"=w249:refnum<queue>)  [unwired: 7 in, 1 out]
          }
        }
        n184 = call "SRV_Queue Streaming Halt and Restore States.vi"("error in (no error)"=w242, "Commands"=T18[] [{"Command"="CCode", "Data"=variant}], "Control Queue"=w243) -> ()  [unwired: 7 in, 2 out]
        n185 = property on="Show Image" class="Bool (strict)"("DisabledEnum"=T17."Disabled and Grayed Out" ("Disabled")) -> ()  [unwired: 2 in, 2 out]
      }
      event #10 {
        n186 = event-data() -> ()  [unwired: 1 in, 1 out]
        n187 = local read "In Pico"() -> (w254:bool)
        n188 = case shown="True" w254 {
          tunnel: w257 -> [w258 w261]
          tunnel: [w258 w260] -> w255
          tunnel: [_ w259] -> w253
          frame #0 {
          }
          frame #1 {
            n189 = call "SRV_Queue_Enqueue Element.vi"("Command"="Escape" ("name (unnamed)"), "Command-Data Queue"=w261) -> ("error out"=w259:errorcluster, "Command-Data Queue out"=w260:refnum<queue>)  [unwired: 7 in, 1 out]
          }
        }
        n190 = call "SRV_Queue_Enqueue Element.vi"("error in (no error)"=w253, "Command"="RunCode" ("name (unnamed)"), "Command-Data Queue"=w255) -> ()  [unwired: 6 in, 3 out]
      }
      event #11 {
        n191 = event-data() -> ()  [unwired: 1 in, 1 out]
        n192 = local read "In Pico"() -> (w265:bool)
        n193 = case shown="True" w265 {
          tunnel: w268 -> [w269 w272]
          tunnel: [w269 w271] -> w266
          tunnel: [_ w270] -> w264
          frame #0 {
          }
          frame #1 {
            n194 = call "SRV_Queue_Enqueue Element.vi"("Command"="Escape" ("name (unnamed)"), "Command-Data Queue"=w272) -> ("error out"=w270:errorcluster, "Command-Data Queue out"=w271:refnum<queue>)  [unwired: 7 in, 1 out]
          }
        }
        n195 = call "SRV_Queue_Enqueue Element.vi"("error in (no error)"=w264, "Command"="ViewCode" ("name (unnamed)"), "Command-Data Queue"=w266) -> ()  [unwired: 6 in, 3 out]
      }
      event #12 {
        n196 = event-data() -> ()  [unwired: 1 in, 1 out]
        n197 = local read "In Pico"() -> (w276:bool)
        n198 = case shown="True" w276 {
          tunnel: w279 -> [w280 w283]
          tunnel: [w280 w282] -> w277
          tunnel: [_ w281] -> w275
          frame #0 {
          }
          frame #1 {
            n199 = call "SRV_Queue_Enqueue Element.vi"("Command"="Escape" ("name (unnamed)"), "Command-Data Queue"=w283) -> ("error out"=w281:errorcluster, "Command-Data Queue out"=w282:refnum<queue>)  [unwired: 7 in, 1 out]
          }
        }
        n200 = call "SRV_Queue_Enqueue Element.vi"("error in (no error)"=w275, "Command"="ImageManip" ("name (unnamed)"), "Command-Data Queue"=w277) -> ()  [unwired: 6 in, 3 out]
      }
      event #13 {
        n201 = event-data() -> ()  [unwired: 1 in, 5 out]
        n202 = local read "In Pico"() -> (w287:bool)
        n203 = case shown="True" w287 {
          tunnel: w290 -> [w291 w294]
          tunnel: [w291 w293] -> w288
          tunnel: [_ w292] -> w286
          frame #0 {
          }
          frame #1 {
            n204 = call "SRV_Queue_Enqueue Element.vi"("Command"="Escape" ("name (unnamed)"), "Command-Data Queue"=w294) -> ("error out"=w292:errorcluster, "Command-Data Queue out"=w293:refnum<queue>)  [unwired: 7 in, 1 out]
          }
        }
        n205 = call "SRV_Queue_Enqueue Element.vi"("error in (no error)"=w286, "Command"="Segment" ("name (unnamed)"), "Command-Data Queue"=w288) -> ()  [unwired: 6 in, 3 out]
      }
      event #14 {
        n206 = event-data() -> ()  [unwired: 1 in, 1 out]
        n207 = local read "In Pico"() -> (w298:bool)
        n208 = case shown="True" w298 {
          tunnel: w301 -> [w302 w305]
          tunnel: [w302 w304] -> w299
          tunnel: [_ w303] -> w297
          frame #0 {
          }
          frame #1 {
            n209 = call "SRV_Queue_Enqueue Element.vi"("Command"="Escape" ("name (unnamed)"), "Command-Data Queue"=w305) -> ("error out"=w303:errorcluster, "Command-Data Queue out"=w304:refnum<queue>)  [unwired: 7 in, 1 out]
          }
        }
        n210 = call "SRV_Queue_Enqueue Element.vi"("error in (no error)"=w297, "Command"="Threshold" ("name (unnamed)"), "Command-Data Queue"=w299) -> ()  [unwired: 6 in, 3 out]
      }
      event #15 {
        n211 = event-data() -> ()  [unwired: 1 in, 1 out]
        n212 = call "SRV_Queue_Enqueue Element.vi"("Command"="Escape" ("name (unnamed)"), "Command-Data Queue"=w308) -> ()  [unwired: 7 in, 3 out]
      }
      event #16 {
        n213 = event-data() -> ()  [unwired: 1 in, 1 out]
        n214 = call "SRV_Queue_Enqueue Element.vi"("Command"="Version" ("name (unnamed)"), "Command-Data Queue"=w311) -> ()  [unwired: 7 in, 3 out]
      }
      event #17 {
        n215 = event-data() -> ()  [unwired: 1 in, 1 out]
        n216 = call "SRV_Queue_Enqueue Element.vi"("Command"="Clear" ("name (unnamed)"), "Command-Data Queue"=w314) -> ()  [unwired: 7 in, 3 out]
      }
      event #18 {
        n217 = event-data() -> ()  [unwired: 1 in, 5 out]
        n218 = call "SRV_Queue_Enqueue Element.vi"("error in (no error)"=w318, "Data"="Show Image", "Command"="Video Streaming" ("element"), "Command-Data Queue"=w320) -> ("error out"=w317:errorcluster)  [unwired: 5 in, 2 out]
      }
      event #19 {
        n219 = event-data() -> ()  [unwired: 1 in, 5 out]
        n220 = call "SRV_Queue_Enqueue Element.vi"("error in (no error)"=w322, "Command"="Edit Motors Config" ("name (unnamed)"), "Command-Data Queue"=w324) -> ("error out"=w321:errorcluster)  [unwired: 6 in, 2 out]
      }
      event #20 {
        n221 = event-data() -> ()  [unwired: 1 in, 5 out]
        n222 = call "SRV_Queue_Enqueue Element.vi"("error in (no error)"=w326, "Command"="Edit Sensors Config" ("name (unnamed)"), "Command-Data Queue"=w328) -> ("error out"=w325:errorcluster)  [unwired: 6 in, 2 out]
      }
      event #21 {
        n223 = event-data() -> ()  [unwired: 1 in, 5 out]
        n224 = call "SRV_Queue_Enqueue Element.vi"("error in (no error)"=w330, "Command"="Edit System Config" ("name (unnamed)"), "Command-Data Queue"=w332) -> ("error out"=w329:errorcluster)  [unwired: 6 in, 2 out]
      }
      event #22 {
        n225 = event-data() -> ("NewVal"=w335:bool, "CtlRef"=w342:refnum<vi>)  [unwired: 1 in]
        n226 = property class="Bool (strict)"(reference=w342, error in=w341) -> (error out=w340:errorcluster, "Label.Text"=w338:string)  [unwired: 1 out]
        n227 = Search 1D Array(1D array=w339, element=w338) -> (index of element=w336:i32)  [unwired: 1 in]
        n228 = Bundle By Name(cluster=T21 {"Button NewVal"=FALSE, "Button Index"=-1} ("Button Event Data"), "Button NewVal"=w335, "Button Index"=w336) -> (w333:T21)
        n229 = call "SRV_Queue_Enqueue Element.vi"("error in (no error)"=w340, "Data"=w333, "Command"="Button Value Change" ("name (unnamed)"), "Command-Data Queue"=w344) -> ("error out"=w343:errorcluster)  [unwired: 5 in, 2 out]
      }
    }
    "i1" <- w177
  }
  n230 = disable-structure shown="Disabled" {
    frame #0 {
      # "These are here so that they are included in a Save for Distribution."
      n231 = call "SRV_Sensor View Tab GUI_DEFAULT.vit"() -> ()  [unwired: 11 in, 1 out]
      n232 = call "SRV_TOOL_Edit Configs_MAIN.vi"() -> ()  [unwired: 11 in, 1 out]
    }
    frame #1 {
    }
  }
  n233 = call "SRV_PM_Receive State Machine.vi"("Cancelled?"=w108, "error in (no error)"=w143, "SRV_Packets queue"=w114, "TCP Read semaphore"=w109, "SRV IP Address"=w110) -> ("error out"=w128:errorcluster)  [unwired: 6 in]
  n234 = call "SRV_Watchdog State Machine.vi"("Cancelled?"=w108, "error in (no error)"=w111, "TCP Read semaphore"=w109, "SRV IP Address"=w110) -> ("error out"=w107:errorcluster)  [unwired: 7 in]
  n235 = while {
    tunnel: w138 -> [w359]
    shift-right: [w352] -> w140
    shift-left: w132 -> [w348]
    shift-right: [w350] -> w127
    shift-left: w135 -> [w365]
    tunnel: w109 -> [w361]
    tunnel: w141 -> [w356]
    tunnel: w142 -> [w353]
    tunnel: w114 -> [w345]
    i -> [w357]
    stop <- w362 stop-if-true
    # "SRV Packets Q"
    # "TCP Read sema"
    # "# IMJ Requests sema"
    # "# IMJ Requests ref"
    # "local data"
    # "Control Q"
    n236 = call "SRV_Queue_Dequeue Element.vi"("timeout in ms (-1)"=500, "error in (no error)"=w348, "Command-Data Queue"=w359) -> ("error out"=w347:errorcluster, "Data"=w354:variant, "Command"=w355:string, "Command-Data Queue out"=w358:refnum<queue>)  [unwired: 3 in, 2 out]
    n237 = case shown="\"Initialize\"" w355 {
      selector: w355 -> [w391 _ w446 _ _ _ _ _ _ _ _ _ _ _ _ _ _ _ _ _ _ _ _ _ _ _ _ _ _ _ _ w932 _ _]
      tunnel: [_ _ _ _ _ _ _ _ _ _ _ _ _ _ _ _ _ _ _ _ _ _ _ _ _ _ _ _ _ _ _ _ _ TRUE] -> w362
      tunnel: w354 -> [_ _ _ _ _ _ _ _ _ _ _ _ _ w636 _ _ _ _ _ _ _ _ _ _ _ _ _ w893 _ _ _ _ _ _]
      tunnel: w358 -> [w382 _ w434 _ w526 w538 _ _ _ _ _ _ _ _ _ _ _ _ _ _ _ _ w804 _ w841 w854 w867 _ _ _ w926 _ _ w957]
      tunnel: w347 -> [w392 w421 w448 w489 w522 w528 w560 w576 w592 w601 w608 w616 w622 w635 w656 w662 w685 w720 w769 w779 w790 w797 w801 w824 w845 w858 w871 w892 w908 w919 w925 w929 w940 w964]
      tunnel: w365 -> [w380 w413 w431 w490 w524 w529 w556 w572 w587 w594 w603 w610 w617 w624 w653 w657 w677 w710 w761 w774 w785 w792 w802 w819 w839 w852 w865 w898 w907 w918 w928 w934 w935 w956]
      tunnel: [w379 w420 w437 w493 w524 w529 w556 w571 w589 w596 w605 w612 w619 w638 w653 w659 w678 w712 w762 w776 w787 w794 w802 w821 w839 w852 w865 w897 w907 w917 w928 w934 w937 w956] -> w350
      tunnel: w361 -> [_ _ _ _ _ _ _ _ _ _ _ _ _ _ _ _ w696 w733 w749 _ _ _ _ _ _ _ _ _ _ _ _ _ _ _]
      tunnel: w356 -> [_ _ _ _ _ _ w558 _ _ _ _ _ _ _ _ _ w687 w722 _ _ _ _ _ _ _ _ _ _ _ _ _ _ _ w959]
      tunnel: w353 -> [_ _ _ _ _ _ w557 _ _ _ _ _ _ _ _ _ w682 w716 _ _ _ _ _ _ _ _ _ _ _ _ _ _ _ w960]
      tunnel: [w381 w416 w442 w495 w525 w539 w554 w575 w591 w598 w607 w615 w621 w639 w655 w661 w695 w717 w756 w778 w789 w796 w800 w823 w842 w855 w868 w894 w904 w919 w922 w931 w939 w948] -> w346
      tunnel: w345 -> [_ _ _ _ _ _ _ _ _ _ _ _ _ _ _ _ _ _ _ _ _ _ _ _ _ _ _ _ _ _ _ _ _ w952]
      frame #0 {
        w378 = FALSE ("In Pico")
        n238 = Unbundle By Name(w380) -> ("Main Controller ref"=w371:refnum<vi>, "Default Config Dir"=w375:path, "Status"=w383:refnum<vi>)
        n239 = call "SRV_Update Status Indicator.vi"("Status ref"=w383, "Status"=w391, "error in (no error)"=w392) -> ("error out"=w376:errorcluster)  [unwired: 11 in, 1 out]
        n240 = call "SRV_SysConfig Initialization Routine.vi"("Config Dir"=w375, "error in (no error)"=w376) -> ("SystemConfig Filepath"=w367:path, "Cancelled?"=w374:bool, "Sys Config Name"=w373:string, "error out"=w369:errorcluster)  [unwired: 8 in, 2 out]
        "System Config" <- w373
        n241 = local write "Expand-Collapse"(FALSE ("Expand-Collapse")) -> ()
        n242 = call "SRV_VIG_System Config Name.vi"("Method (Get)"=enum16{"Get", "Set"}."Set", "SystemConfig Filepath"=w367, "System Config Name"=w373) -> ()  [unwired: 6 in, 3 out]
        n243 = property on="Cover" class="Bool (strict)"("Visible"=FALSE) -> ()  [unwired: 2 in, 2 out]
        n244 = local write "Plan"(T5."Nothing" ("Plan")) -> ()
        n245 = call "SRV_Get OS Version.vi"("error in (no error)"=w369) -> ("Equal or Newer Version?"=w370:bool, "error out"=w368:errorcluster)  [unwired: 12 in, 1 out]
        n246 = property on="SRV IP Address" class="Str"("DisabledEnum"=T17."Disabled" ("Disabled")) -> ()  [unwired: 2 in, 2 out]
        n247 = local write "Tab Control"(u32 0) -> ()
        n248 = call "SRV_Fit VI window to Largest Dec__ogtk.vi"("border spacing (2 px)"=0, "VI Ref (calling VI)"=w371) -> ("error out"=w388:errorcluster, "dup VI Ref"=w389:refnum<vi>)  [unwired: 4 in]
        n249 = case "Cancelled?" shown="False" w374 {
          selector: w374 -> [_ w404]
          tunnel: w382 -> [w399 w409]
          tunnel: [w398 w405] -> w381
          tunnel: w368 -> [w397 w410]
          tunnel: w378 -> [_ w408]
          tunnel: string[] ["InitMotors", "InitTCP", "Open Sensor View"] -> [w396 _]
          frame #0 {
            n250 = for {
              tunnel: w399 -> [w403]
              shift-right: [w402] -> w398
              shift-left: w397 -> [w401]
              tunnel: w396 -> [w400] mode=indexing
              n251 = call "SRV_Queue_Enqueue Element.vi"("error in (no error)"=w401, "Command"=w400, "Command-Data Queue"=w403) -> ("error out"=w402:errorcluster)  [unwired: 6 in, 2 out]
            }
          }
          frame #1 {
            n252 = call "SRV_Queue Shutdown States.vi"("error in (no error)"=w410, "In Pico"=w408, "Control Queue"=w409) -> ("error out"=w406:errorcluster)  [unwired: 7 in, 1 out]
            n253 = call "SRV_SRV_Loops Notifier.vi"("Notifier Methods"=SRV_SRV_Loops_Notifier_Methods."Send Notification", "error in (no error)"=w406, "Cancelled? (F)"=w404) -> ("error out"=w405:errorcluster)  [unwired: 7 in, 1 out]
          }
        }
        n254 = Bundle By Name(cluster=w380, "System Config Name"=w373, "VISTA or Later?"=w370) -> (w379:T8)
        n255 = call "SRV_Update Main Window Title and Open Window.vi"("VI ref"=w389, "error in (no error)"=w388) -> ()  [unwired: 12 in, 2 out]
        n256 = local write "Movie Mode"(FALSE ("Movie")) -> ()
        "Number of IMJ Requests" <- 0 ("Number of IMJ Requests")
        "In Pico" <- w378
        "Replies" <- ""
        "InPico State Change" <- w378
      }
      frame #1 {
        n257 = call "SRV_Main Config Paths.vi"("local data"=w413) -> ("local data dup"=w412:T8, "MotorsConfig Filepath"=w414:path)  [unwired: 8 in, 5 out]
        n258 = Unbundle By Name(w412) -> ("button refs"=w411:refnum<vi>[], "false refs"=w418:refnum<vi>[], "true refs"=w417:refnum<vi>[])
        n259 = call "SRV_Check File Exists with Dialog.vi"("Filepath"=w414, "File Type"="Motor Config File", "error in (no error)"=w421) -> ("Filepath dup"=w422:path, "File Exists?"=w415:bool, "error out"=w423:errorcluster)  [unwired: 10 in]
        n260 = call "SRV_Initialize Motor Buttons.vi"("Motors Config File Path"=w422, "button refs"=w411, "false refs"=w418, "true refs"=w417, "Init from File (F)"=w415, "error in (no error)"=w423) -> ("Motor Control Config"=w419:T9[], "error out"=w416:errorcluster)  [unwired: 8 in]
        n261 = Bundle By Name(cluster=w413, "Motor Control Config"=w419) -> (w420:T8)
      }
      frame #2 {
        n262 = Unbundle By Name(w431) -> ("Status"=w447:refnum<vi>)
        n263 = call "SRV_Main Config Paths.vi"("local data"=w431) -> ("SystemConfig Filepath"=w430:path)  [unwired: 8 in, 6 out]
        n264 = call "SRV_Update Status Indicator.vi"("Status ref"=w447, "Status"=w446, "error in (no error)"=w448) -> ("Status ref out"=w432:refnum<vi>, "error out"=w428:errorcluster)  [unwired: 11 in]
        n265 = call "SRV_Read System Config File.vi"("System Config File Path"=w430, "error in (no error)"=w428) -> ("System Config"=w429:T26, "error out"=w427:errorcluster)  [unwired: 10 in, 2 out]
        n266 = call "SRV_Init_TCP Comm Loop.vi"("error in (no error)"=w427, "System Config File Path in"=w430) -> ("error out"=w440:errorcluster, "Cancelled?"=w435:bool, "SRV IP Address out"=w439:string, "connection ID"=w441:refnum<k5>)  [unwired: 6 in]
        n267 = Unbundle By Name(w429) -> ("Enable Diagnostic Log"=w426:bool)
        n268 = case "Cancelled?" shown="False" w435 {
          tunnel: w441 -> [w456 w474]
          tunnel: w440 -> [w455 w475]
          tunnel: [w454 w474] -> w436
          tunnel: [w453 w475] -> w438
          frame #0 {
            n269 = call "SRV_PM_VIG_Packet Mode.vi"() -> ("Packet Mode Style"=w452:T19)  [unwired: 15 in]
            n270 = case shown="\"New PM\"" w452 {
              tunnel: w456 -> [w464 w471]
              tunnel: w455 -> [w463 w472]
              tunnel: [w462 w468] -> w454
              tunnel: [w461 w467] -> w453
              frame #0 {
                n271 = call "CameraSetup.vi"("error in (no error)"=w463, "Task"=T22."Disable", "SRV In"=w464) -> ("error out"=w459:errorcluster, "SRV Out"=w458:refnum<k5>)  [unwired: 7 in]
                n272 = call "SRV_Write_Comm.vi"("error in (no error)"=w459, "Command Sent"="V", "SRV In"=w458) -> ("error out"=w461:errorcluster, "SRV Out"=w462:refnum<k5>)  [unwired: 6 in, 1 out]
              }
              frame #1 {
                n273 = call "SRV_PM_App Initializaton Routine.vi"("Packet Mode Enable (T)"=TRUE, "Read Response (F)"=FALSE, "error in (no error)"=w472, "connection ID"=w471) -> ("error out"=w466:errorcluster, "connection ID out"=w469:refnum<k5>)  [unwired: 4 in, 2 out]
                n274 = call "CameraSetup.vi"("error in (no error)"=w466, "Task"=T22."Disable", "SRV In"=w469) -> ("error out"=w467:errorcluster, "SRV Out"=w468:refnum<k5>)  [unwired: 7 in]
              }
            }
          }
          frame #1 {
          }
        }
        n275 = flat-sequence {
          tunnel: w426 -> [w450]
          tunnel: [SRV_SRV_Loops_Notifier_Methods."Send Notification" ("Notifier Methods")] -> w425
          frame #0 {
            n276 = call "SRV_VIG_System Config-Enable Diagnostic Logging.vi"("Enable Diagnostic Log"=w450, "Method (Get)"=enum16{"Get", "Set"}."Set") -> ()  [unwired: 13 in, 1 out]
          }
        }
        n277 = flat-sequence {
          tunnel: w439 -> [w476]
          tunnel: w436 -> [w478]
          tunnel: w438 -> [w477]
          tunnel: [w477] -> w433
          frame #0 {
            "SRV Out" <- w478
            "SRV IP Address" <- w476
          }
        }
        n278 = call "SRV_Update Status Indicator.vi"("Status ref"=w432, "error in (no error)"=w433) -> ("error out"=w445:errorcluster)  [unwired: 12 in, 1 out]
        n279 = case "Cancelled?" shown="True" w435 {
          selector: w435 -> [w479 w485]
          tunnel: w445 -> [w482 w488]
          tunnel: [w481 w487] -> w444
          tunnel: w434 -> [w480 w486]
          tunnel: [w479 w485] -> w443
          frame #0 {
            n280 = call "SRV_Queue_Enqueue Element.vi"("error in (no error)"=w482, "Command"="Version" ("element"), "Command-Data Queue"=w480) -> ("error out"=w481:errorcluster)  [unwired: 6 in, 2 out]
          }
          frame #1 {
            n281 = local read "In Pico"() -> (w484:bool)
            n282 = call "SRV_Queue Shutdown States.vi"("error in (no error)"=w488, "In Pico"=w484, "Control Queue"=w486) -> ("error out"=w487:errorcluster)  [unwired: 7 in, 1 out]
          }
        }
        n283 = call "SRV_SRV_Loops Notifier.vi"("Notifier Methods"=w425, "error in (no error)"=w444, "Cancelled? (F)"=w443) -> ("error out"=w442:errorcluster)  [unwired: 7 in, 1 out]
        n284 = Bundle By Name(cluster=w431, "SRV"=w436) -> (w437:T8)
      }
      frame #3 {
        n285 = call "SRV_Shutdown Flag.vi"() -> ("Shutdown Flag out"=w491:bool)  [unwired: 14 in, 1 out]
        n286 = case "Shutdown Flag set?" shown="False" w491 {
          tunnel: [w508 _] -> w494
          tunnel: [w507 _] -> w492
          tunnel: w490 -> [w500 _]
          frame #0 {
            n287 = Unbundle By Name(w500) -> ("SRV"=w503:refnum<k5>, "VISTA or Later?"=w498:bool, "Main Controller ref"=w496:refnum<vi>)
            n288 = call "SRV_Main Config Paths.vi"("local data"=w500) -> ("SystemConfig Filepath"=w499:path, "SensorsConfig Filepath"=w504:path)  [unwired: 8 in, 5 out]
            n289 = local read "Expand-Collapse"() -> (w497:bool)
            n290 = call "SRV_Get Sensor Window Filepath.vi"("System Config File Path"=w499) -> ("error out"=w501:errorcluster, "Sensor Window Filepath"=w502:path)  [unwired: 9 in]
            n291 = call "SRV_Update Streaming States VIG.vi"("Enabled"=TRUE, "Streaming Modes"=SRV_Streaming_Modes."Sensors") -> ()  [unwired: 14 in]
            n292 = call "SRV_Launch Sensor View Tab GUI.vi"("VI Path"=w502, "Sensors Config File Path"=w504, "SRV In"=w503, "Vista or Later?"=w498, "error in (no error)"=w501, "Main Controller ref"=w496, "Expand-Collapse"=w497) -> ("VI refnum out"=w507:refnum<vi>, "error out"=w508:errorcluster)  [unwired: 6 in, 1 out]
          }
          frame #1 {
          }
        }
        n293 = Bundle By Name(cluster=w490, "Sensor View ref"=w492) -> (w493:T8)
        n294 = Select(t=w489, s=w489, f=w494) -> (s? t:f=w495:errorcluster)
      }
      frame #4 {
        n295 = Unbundle By Name(w524) -> ("Status"=w516:refnum<vi>, "VISTA or Later?"=w509:bool, "Sensor View ref"=w523:refnum<vi>, "Main Controller ref"=w521:refnum<vi>)
        n296 = call "SRV_Manage Window Sizes.vi"("Sensor View ref"=w523, "Vista or Later?"=w509, "Main Controller ref"=w521, "Expand-Collapse"="Expand-Collapse", "error in (no error)"=w522) -> ("error out"=w520:errorcluster)  [unwired: 10 in]
        n297 = Select(t="Collapse to hide tabs..." ("Tip Strip"), s="Expand-Collapse", f="Expand to show tabs..." ("Tip Strip")) -> (s? t:f=w519:string)
        n298 = Select(t=T24 {"Width"=1180, "Height"=25} ("Size"), s="Expand-Collapse", f=T24 {"Width"=412, "Height"=25} ("Size")) -> (s? t:f=w514:T24)
        n299 = property on="Expand-Collapse" class="Bool (strict)"(error in=w520, "TipStrip"=w519) -> (error out=w512:errorcluster)  [unwired: 1 in, 1 out]
        n300 = property class="Str"(reference=w516, error in=w512, "Size"=w514) -> (error out=w511:errorcluster)  [unwired: 1 out]
        n301 = call "SRV_Queue_Enqueue Element.vi"("error in (no error)"=w511, "Command"="Manage InPico State" ("element"), "Command-Data Queue"=w526) -> ("error out"=w525:errorcluster)  [unwired: 6 in, 2 out]
      }
      frame #5 {
        # "The boolean logic here is all about getting one more PicoC Buffer Read after the In Pico light goes off."
        n302 = local read "InPico State Change"() -> (w535:bool)
        n303 = local read "In Pico"() -> (w532:bool)
        n304 = call "SRV_In PicoC State Change.vi"("In Pico"=w532, "InPico State Change"=w535) -> ("Read PicoC Buffer?"=w530:bool, "InPico State Change out"=w534:bool)  [unwired: 8 in]
        n305 = call "SRV_Manage Time Interval for Read.vi"("Some State"=w532, "Read Interval (1000 ms)"=u32 1000) -> ("Time to Read?"=w537:bool, "State Change?"=w533:bool)  [unwired: 12 in]
        n306 = Compound Arithmetic op=OR(w530, w532, w533) -> (w531:bool)
        n307 = local write "InPico State Change"(w534) -> ()
        n308 = case shown="True" w531 {
          tunnel: w528 -> [w540 w547]
          tunnel: [w540 w546] -> w539
          tunnel: w538 -> [_ w545]
          tunnel: w537 -> [_ w543]
          tunnel: w533 -> [_ w544]
          tunnel: w530 -> [_ w542]
          frame #0 {
          }
          frame #1 {
            n309 = Compound Arithmetic op=OR(w542, w543, w544) -> (w541:bool)
            n310 = case shown="True" w541 {
              tunnel: w547 -> [w548 w552]
              tunnel: [w548 w551] -> w546
              tunnel: w545 -> [_ w550]
              frame #0 {
              }
              frame #1 {
                n311 = call "SRV_Queue_Enqueue Element.vi"("error in (no error)"=w552, "Command"="Read PicoC Buffer", "Command-Data Queue"=w550) -> ("error out"=w551:errorcluster)  [unwired: 6 in, 2 out]
              }
            }
          }
        }
      }
      frame #6 {
        w553 = FALSE  # Show Image
        n312 = Unbundle By Name(w556) -> ("SRV"=w555:refnum<k5>)
        n313 = Not(x=w553) -> (.not. x?=w559:bool)
        n314 = property on="Cover" class="Bool (strict)"("Visible"=w559) -> ()  [unwired: 2 in, 2 out]
        n315 = case shown="True" w553 {
          tunnel: w560 -> [w561 w566]
          tunnel: [w561 w568] -> w554
          tunnel: w555 -> [_ w567]
          tunnel: w558 -> [_ w564]
          tunnel: w557 -> [_ w562]
          frame #0 {
          }
          frame #1 {
            n316 = call "SRV_Number of IMJ Requests Methods.vi"("Number of IMJ Requests ref"=w564, "semaphore ref"=w562, "error in (no error)"=w566, "Number of IMJ Requests Methods (Read)"=SRV_Number_of_IMJ_Requests_Methods."Increment" ("Number of IMJ Requests Methods")) -> ("error out"=w565:errorcluster)  [unwired: 7 in, 4 out]
            n317 = call "SRV_Write_Comm.vi"("error in (no error)"=w565, "Command Sent"="I", "SRV In"=w567) -> ("error out"=w568:errorcluster)  [unwired: 6 in, 2 out]
          }
        }
      }
      frame #7 {
        n318 = Unbundle By Name(w572) -> ("SRV"=w573:refnum<k5>)
        n319 = case shown="Default" "Direct Command to Send" {
          selector: "Direct Command to Send" -> [_ w579]
          tunnel: w573 -> [w577 w584]
          tunnel: [w577 w583] -> w570
          tunnel: w576 -> [w578 w582]
          tunnel: [w578 w581] -> w575
          frame #0 {
          }
          frame #1 {
            n320 = call "SRV_Write_Comm.vi"("error in (no error)"=w582, "Command Sent"=w579, "SRV In"=w584) -> ("error out"=w581:errorcluster, "Command Sent dup"=w580:string, "SRV Out"=w583:refnum<k5>)  [unwired: 6 in]
            n321 = case shown="\"!\", \"Q\"" w580 {
              frame #0 {
              }
              frame #1 {
                w585 = TRUE ("In Pico")
                n322 = local write "InPico State Change"(w585) -> ()
                n323 = local write "In Pico"(w585) -> ()
              }
            }
          }
        }
        n324 = Bundle By Name(cluster=w572, "SRV"=w570) -> (w571:T8)
      }
      frame #8 {
        w590 = TRUE ("In Pico")
        n325 = Unbundle By Name(w587) -> ("SRV"=w588:refnum<k5>)
        n326 = call "SRV_Write_Comm.vi"("error in (no error)"=w592, "Command Sent"="Q" ("name (unnamed)"), "SRV In"=w588) -> ("error out"=w591:errorcluster, "SRV Out"=w586:refnum<k5>)  [unwired: 6 in, 1 out]
        n327 = local write "In Pico"(w590) -> ()
        n328 = local write "InPico State Change"(w590) -> ()
        n329 = Bundle By Name(cluster=w587, "SRV"=w586) -> (w589:T8)
      }
      frame #9 {
        # "Wait here to avoid enqueuing more \"I\" (Grab Image) before this has a chance to read all the code in the lower loop. Without waiting, you get binary jpeg info along with the read code in the Replies window.\n\nThis is not an elegant solution...should code semaphore type functionality but what is trickier than with the XModem code is the verification that you are done reading the C code comes in the lower loop.\n\nIs there some sort of term char that goes with the message that we can read until we find??"
        n330 = Unbundle By Name(w594) -> ("SRV"=w597:refnum<k5>)
        n331 = call "SRV_Write_Comm.vi"("error in (no error)"=w601, "Command Sent"="zd" ("name (unnamed)"), "SRV In"=w597) -> ("error out"=w599:errorcluster, "SRV Out"=w595:refnum<k5>)  [unwired: 6 in, 1 out]
        n332 = call "SRV_Wait (ms)+.vi"("milliseconds to wait"=u32 500 ("Delay (ms)"), "error in (no error)"=w599) -> ("error out"=w598:errorcluster)  [unwired: 12 in, 1 out]
        n333 = Bundle By Name(cluster=w594, "SRV"=w595) -> (w596:T8)
      }
      frame #10 {
        w609 = FALSE ("Enable?")
        n334 = Unbundle By Name(w603) -> ("SRV"=w606:refnum<k5>)
        n335 = local write "In Pico"(w609) -> ()
        n336 = call "PicoC_Mode.vi"("error in (no error)"=w608, "Enable?"=w609, "SRV In"=w606) -> ("error out"=w607:errorcluster, "SRV Out"=w604:refnum<k5>)  [unwired: 7 in]
        n337 = Bundle By Name(cluster=w603, "SRV"=w604) -> (w605:T8)
      }
      frame #11 {
        w614 = TRUE ("Enable?")
        # "Never gets here."
        n338 = Unbundle By Name(w610) -> ("SRV"=w613:refnum<k5>)
        n339 = local write "In Pico"(w614) -> ()
        n340 = local write "InPico State Change"(w614) -> ()
        n341 = call "PicoC_Mode.vi"("error in (no error)"=w616, "Enable?"=w614, "SRV In"=w613) -> ("error out"=w615:errorcluster, "SRV Out"=w611:refnum<k5>)  [unwired: 7 in]
        n342 = Bundle By Name(cluster=w610, "SRV"=w611) -> (w612:T8)
      }
      frame #12 {
        n343 = Unbundle By Name(w617) -> ("SRV"=w620:refnum<k5>)
        n344 = call "SRV_Write_Comm.vi"("error in (no error)"=w622, "Command Sent"="V", "SRV In"=w620) -> ("error out"=w621:errorcluster, "SRV Out"=w618:refnum<k5>)  [unwired: 6 in, 1 out]
        n345 = Bundle By Name(cluster=w617, "SRV"=w618) -> (w619:T8)
      }
      frame #13 {
        w632 = "$v2"  # Turn Video Streaming Off
        w633 = "$v1"  # Turn Video Streaming On
        n346 = Unbundle By Name(w624) -> ("SRV"=w629:refnum<k5>)
        n347 = Variant To Data(error in=w635, Variant=w636, type=FALSE ("Video Streaming")) -> (error out=w625:errorcluster, data=w626:bool)
        n348 = case shown="True" w626 {
          tunnel: w629 -> [w640 w650]
          tunnel: [w640 w649] -> w628
          tunnel: w625 -> [w641 w645]
          tunnel: [w641 w648] -> w627
          tunnel: w624 -> [_ w642]
          frame #0 {
          }
          frame #1 {
            n349 = call "SRV_Main Config Paths.vi"("local data"=w642) -> ("SystemConfig Filepath"=w643:path)  [unwired: 8 in, 6 out]
            n350 = call "SRV_Read System Config File.vi"("System Config File Path"=w643, "error in (no error)"=w645) -> ("System Config"=w646:T26, "error out"=w644:errorcluster)  [unwired: 10 in, 2 out]
            n351 = Unbundle By Name(w646) -> ("Video Stream Rate Period (ms)"=w651:u32)
            n352 = call "SRV_Build Video Stream Rate Command.vi"("Video Stream Rate Period (ms)"=w651) -> ("Command String"=w647:string)  [unwired: 9 in, 1 out]
            n353 = call "SRV_Write_Comm.vi"("error in (no error)"=w644, "Command Sent"=w647, "SRV In"=w650) -> ("error out"=w648:errorcluster, "SRV Out"=w649:refnum<k5>)  [unwired: 6 in, 1 out]
          }
        }
        n354 = Select(t=w633, s=w626, f=w632) -> (s? t:f=w631:string)
        n355 = call "SRV_Write_Comm.vi"("error in (no error)"=w627, "Command Sent"=w631, "SRV In"=w628) -> ("error out"=w639:errorcluster, "SRV Out"=w637:refnum<k5>)  [unwired: 6 in, 1 out]
        n356 = call "SRV_Update Streaming States VIG.vi"("Enabled"=w626, "Streaming Modes"=SRV_Streaming_Modes."Video") -> ()  [unwired: 14 in]
        n357 = Bundle By Name(cluster=w624, "SRV"=w637) -> (w638:T8)
      }
      frame #14 {
        n358 = Unbundle By Name(w653) -> ("Replies"=w652:refnum<vi>)
        n359 = call "SRV_Update Replies Indicator.vi"("Replies ref"=w652, "Text to Append"="xXxClearRepliesxXx", "error in (no error)"=w656) -> ("error out"=w655:errorcluster)  [unwired: 11 in, 1 out]
      }
      frame #15 {
        n360 = Unbundle By Name(w657) -> ("SRV"=w660:refnum<k5>)
        n361 = call "SRV_Write_Comm.vi"("error in (no error)"=w662, "Command Sent"="*B\r", "SRV In"=w660) -> ("error out"=w661:errorcluster, "SRV Out"=w658:refnum<k5>)  [unwired: 6 in, 1 out]
        n362 = Bundle By Name(cluster=w657, "SRV"=w658) -> (w659:T8)
      }
      frame #16 {
        n363 = Unbundle By Name(w677) -> ("Replies"=w676:refnum<vi>, "SRV"=w667:refnum<k5>, "Status"=w675:refnum<vi>)
        n364 = call "SRV_Update Status Indicator.vi"("Status ref"=w675, "Status"="Waiting to load C Code...", "error in (no error)"=w685) -> ("Status ref out"=w684:refnum<vi>, "error out"=w686:errorcluster)  [unwired: 11 in]
        n365 = call "SRV_Wait for Zero IMJ Requests.vi"("Number of IMJ Requests ref"=w687, "#IMJ semaphore ref"=w682, "error in (no error)"=w686) -> ("error out"=w688:errorcluster)  [unwired: 10 in, 2 out]
        n366 = call <vilib>:"Acquire Semaphore.vi"("error in (no error)"=w688, "semaphore"=w696) -> ("error out"=w691:errorcluster, "semaphore out"=w694:T20)  [unwired: 3 in, 1 out]
        n367 = call "SRV_Update Status Indicator.vi"("Status ref"=w684, "Status"="Loading C Code...", "error in (no error)"=w691, "Delay After Update (0 ms)"=u32 500) -> ("Status ref out"=w690:refnum<vi>, "error out"=w672:errorcluster)  [unwired: 10 in]
        n368 = call "SRV_PM_App Initializaton Routine.vi"("Packet Mode Enable (T)"=FALSE, "Read Response (F)"=TRUE, "error in (no error)"=w672, "connection ID"=w667) -> ("error out"=w671:errorcluster, "connection ID out"=w666:refnum<k5>)  [unwired: 4 in, 2 out]
        n369 = call "SRV_XModem_WriteFile_Comm.vi"("error in (no error)"=w671, "File Contents"="C Code", "SRV In"=w666) -> ("error out"=w670:errorcluster, "SRV Out"=w665:refnum<k5>, "## Reply"=w680:string, "Replies"=w689:string[])  [unwired: 4 in, 1 out]
        n370 = local write "XModem Replies"(w689) -> ()
        n371 = call "SRV_PM_App Initializaton Routine.vi"("Packet Mode Enable (T)"=TRUE, "error in (no error)"=w670, "connection ID"=w665) -> ("error out"=w669:errorcluster, "connection ID out"=w664:refnum<k5>)  [unwired: 5 in, 2 out]
        n372 = call "SRV_Update Status Indicator.vi"("Status ref"=w690, "error in (no error)"=w669) -> ("error out"=w679:errorcluster)  [unwired: 12 in, 1 out]
        n373 = call "SRV_Update Replies Indicator.vi"("Replies ref"=w676, "Text to Append"=w680, "error in (no error)"=w679) -> ("error out"=w681:errorcluster)  [unwired: 11 in, 1 out]
        n374 = Bundle By Name(cluster=w677, "SRV"=w664) -> (w678:T8)
        n375 = call <vilib>:"Release Semaphore.vi"("error in (no error)"=w681, "semaphore"=w694) -> ("error out"=w695:errorcluster)  [unwired: 4 in, 1 out]
      }
      frame #17 {
        n376 = Unbundle By Name(w710) -> ("Replies"=w711:refnum<vi>, "SRV"=w705:refnum<k5>, "Status"=w709:refnum<vi>)
        n377 = call "SRV_Update Status Indicator.vi"("Status ref"=w709, "Status"="Waiting to load firmware...", "error in (no error)"=w720) -> ("Status ref out"=w719:refnum<vi>, "error out"=w721:errorcluster)  [unwired: 11 in]
        n378 = call "SRV_Wait for Zero IMJ Requests.vi"("Number of IMJ Requests ref"=w722, "#IMJ semaphore ref"=w716, "error in (no error)"=w721) -> ("error out"=w723:errorcluster)  [unwired: 10 in, 2 out]
        n379 = call <vilib>:"Acquire Semaphore.vi"("error in (no error)"=w723, "semaphore"=w733) -> ("error out"=w731:errorcluster, "semaphore out"=w732:T20)  [unwired: 3 in, 1 out]
        n380 = call "SRV_Update Status Indicator.vi"("Status ref"=w719, "Status"="Loading Firmware...", "error in (no error)"=w731, "Delay After Update (0 ms)"=u32 250) -> ("Status ref out"=w729:refnum<vi>, "error out"=w708:errorcluster)  [unwired: 10 in]
        n381 = call "SRV_PM_App Initializaton Routine.vi"("Packet Mode Enable (T)"=FALSE, "Read Response (F)"=TRUE, "error in (no error)"=w708, "connection ID"=w705) -> ("error out"=w707:errorcluster, "connection ID out"=w706:refnum<k5>)  [unwired: 4 in, 2 out]
        n382 = Read from Binary File(8:w707, 10:-1 ("count (1)"), 11:"firmware") -> (0:w726:errorcluster, 2:w725:string)  [unwired: 3 in, 2 out]
        n383 = call "SRV_XModem_WriteFile_Comm.vi"("error in (no error)"=w726, "File Contents"=w725, "SRV In"=w706) -> ("error out"=w702:errorcluster, "SRV Out"=w699:refnum<k5>, "## Reply"=w714:string, "Replies"=→"XModem Replies":string[])  [unwired: 4 in, 1 out]
        n384 = call "SRV_PM_App Initializaton Routine.vi"("Packet Mode Enable (T)"=TRUE, "error in (no error)"=w702, "connection ID"=w699) -> ("error out"=w701:errorcluster, "connection ID out"=w698:refnum<k5>)  [unwired: 5 in, 2 out]
        n385 = call "SRV_Update Status Indicator.vi"("Status ref"=w729, "error in (no error)"=w701) -> ("error out"=w713:errorcluster)  [unwired: 12 in, 1 out]
        n386 = call "SRV_Update Replies Indicator.vi"("Replies ref"=w711, "Text to Append"=w714, "error in (no error)"=w713) -> ("error out"=w715:errorcluster)  [unwired: 11 in, 1 out]
        n387 = Bundle By Name(cluster=w710, "SRV"=w698) -> (w712:T8)
        n388 = call <vilib>:"Release Semaphore.vi"("error in (no error)"=w715, "semaphore"=w732) -> ("error out"=w717:errorcluster)  [unwired: 4 in, 1 out]
      }
      frame #18 {
        # "Reboot the blackfin processor.\nThis will not disconnect the radio. It will emerge from the reboot not in packet mode, so read the reboot response on its own and then turn packet mode back on."
        # "copy the firmware from RAM into flash"
        # "Wait for response."
        n389 = Unbundle By Name(w761) -> ("Replies"=w748:refnum<vi>, "SRV"=w763:refnum<k5>, "Status"=w760:refnum<vi>)
        n390 = call "SRV_Update Status Indicator.vi"("Status ref"=w760, "Status"="Copying firmware from RAM into flash (zZ)...", "error in (no error)"=w769, "Delay After Update (0 ms)"=u32 100) -> ("Status ref out"=w765:refnum<vi>, "error out"=w768:errorcluster)  [unwired: 10 in]
        n391 = call "SRV_Write_Comm.vi"("error in (no error)"=w768, "Command Sent"="zZ" ("data in"), "SRV In"=w763) -> ("error out"=w759:errorcluster, "SRV Out"=w772:refnum<k5>)  [unwired: 6 in, 1 out]
        n392 = call "SRV_SRV_zZ Notifier.vi"("Notifier Methods"=SRV_SRV_Loops_Notifier_Methods."Wait on Notification", "error in (no error)"=w759, "timeout in ms (-1)"=10000) -> ("error out"=w754:errorcluster)  [unwired: 8 in]
        n393 = call "SRV_Update Status Indicator.vi"("Status ref"=w765, "Status"="Rebooting the processor ($!)...", "error in (no error)"=w754, "Delay After Update (0 ms)"=u32 250) -> ("Status ref out"=w764:refnum<vi>, "error out"=w753:errorcluster)  [unwired: 10 in]
        n394 = call <vilib>:"Acquire Semaphore.vi"("error in (no error)"=w753, "semaphore"=w749) -> ("error out"=w752:errorcluster, "semaphore out"=w750:T20)  [unwired: 3 in, 1 out]
        n395 = call "SRV_Write_Comm.vi"("error in (no error)"=w752, "Command Sent"="$!" ("data in"), "SRV In"=w772) -> ("error out"=w744:errorcluster, "SRV Out"=w745:refnum<k5>)  [unwired: 6 in, 1 out]
        n396 = call "SRV_Read_Comm.vi"("error in (no error)"=w744, "SRV In"=w745) -> ("error out"=w743:errorcluster, "Data out"=w742:string, "SRV Out"=w738:refnum<k5>)  [unwired: 7 in]
        n397 = call "SRV_Update Replies Indicator.vi"("Replies ref"=w748, "Text to Append"=w742, "error in (no error)"=w743) -> ("Replies ref out"=w737:refnum<vi>, "error out"=w739:errorcluster)  [unwired: 11 in]
        n398 = call "SRV_PM_App Initializaton Routine.vi"("Packet Mode Enable (T)"=TRUE, "Read Response (F)"=TRUE, "error in (no error)"=w739, "connection ID"=w738) -> ("error out"=w736:errorcluster, "connection ID out"=w755:refnum<k5>, "Response"=w735:string)  [unwired: 4 in, 1 out]
        n399 = call "SRV_Update Replies Indicator.vi"("Replies ref"=w737, "Text to Append"=w735, "error in (no error)"=w736) -> ("error out"=w747:errorcluster)  [unwired: 11 in, 1 out]
        n400 = call <vilib>:"Release Semaphore.vi"("error in (no error)"=w747, "semaphore"=w750) -> ("error out"=w751:errorcluster)  [unwired: 4 in, 1 out]
        n401 = call "SRV_Update Status Indicator.vi"("Status ref"=w764, "error in (no error)"=w751) -> ("error out"=w756:errorcluster)  [unwired: 12 in, 1 out]
        n402 = Bundle By Name(cluster=w761, "SRV"=w755) -> (w762:T8)
      }
      frame #19 {
        n403 = Unbundle By Name(w774) -> ("SRV"=w777:refnum<k5>)
        n404 = call "CameraSetup.vi"("error in (no error)"=w779, "Task"=T22."Disable", "SRV In"=w777) -> ("error out"=w780:errorcluster, "SRV Out"=w781:refnum<k5>)  [unwired: 7 in]
        n405 = To Unsigned Word Integer(number="Plan") -> (unsigned 16bit integer=w783:u16)
        n406 = call "CameraSetup.vi"("error in (no error)"=w780, "Task"=w783, "SRV In"=w781) -> ("error out"=w778:errorcluster, "SRV Out"=w775:refnum<k5>)  [unwired: 7 in]
        n407 = Bundle By Name(cluster=w774, "SRV"=w775) -> (w776:T8)
      }
      frame #20 {
        n408 = Unbundle By Name(w785) -> ("SRV"=w788:refnum<k5>)
        n409 = call "CameraThreshold.vi"("error in (no error)"=w790, "Threshold"="Threshold", "SRV In"=w788) -> ("error out"=w789:errorcluster, "SRV Out"=w786:refnum<k5>)  [unwired: 7 in]
        n410 = Bundle By Name(cluster=w785, "SRV"=w786) -> (w787:T8)
      }
      frame #21 {
        n411 = Unbundle By Name(w792) -> ("SRV"=w795:refnum<k5>)
        n412 = To Unsigned Word Integer(number="Bins") -> (unsigned 16bit integer=w798:u16)
        n413 = call "CameraAutoSegmentation.vi"("error in (no error)"=w797, "Bins"=w798, "SRV In"=w795) -> ("error out"=w796:errorcluster, "SRV Out"=w793:refnum<k5>)  [unwired: 7 in]
        n414 = Bundle By Name(cluster=w792, "SRV"=w793) -> (w794:T8)
      }
      frame #22 {
        n415 = local read "Image/Movie Out"() -> (w803:T7)
        n416 = call "GetLastImageName.vi"("Path to folder"="Path to folder") -> ("new path"=w805:path)
        n417 = case shown="True" "Movie Mode" {
          tunnel: w804 -> [_ w815]
          tunnel: w801 -> [w811 w813]
          tunnel: [w811 w812] -> w800
          frame #0 {
          }
          frame #1 {
            # "GrabImage doesn't really work anymore.\nNeed to update to be compatible with Video Streaming mode."
            n418 = call "SRV_Queue_Enqueue Element.vi"("error in (no error)"=w813, "Command"="GrabImage" ("name (unnamed)"), "Command-Data Queue"=w815) -> ("error out"=w814:errorcluster, "Command-Data Queue out"=w816:refnum<queue>)  [unwired: 6 in, 1 out]
            n419 = call "SRV_Queue_Enqueue Element.vi"("error in (no error)"=w814, "Command"="Snap" ("name (unnamed)"), "Command-Data Queue"=w816) -> ("error out"=w812:errorcluster)  [unwired: 6 in, 2 out]
          }
        }
        n420 = Strip Path(path=w805) -> (name=→"Last file name":string)  [unwired: 1 out]
        n421 = disable-structure shown="Disabled" {
          disable-tunnel: w805 -> [w810 _]
          disable-tunnel: w803 -> [w809 _]
          frame #0 {
            n422 = call "LV86_Save JPG.vi"("Path to file"=w810, "Image"=w809) -> ()  [unwired: 1 in, 1 out]
          }
          frame #1 {
          }
        }
      }
      frame #23 {
        n423 = property on="The image" class="Pict"(error in=w824) -> (error out=w825:errorcluster, "Mouse"=w829:T28)  [unwired: 1 in, 1 out]
        n424 = Unbundle By Name(w829) -> ("Mouse Position"=w828:cluster{"X":i32, "Y":i32})
        n425 = local read "Image/Movie Out"() -> (w833:T7)
        n426 = Unbundle By Name(w819) -> ("SRV"=w822:refnum<k5>)
        n427 = Unbundle(w828) -> ("X"=w827:i32, "Y"=w826:i32)
        n428 = call "LV86_Get Pixel Value.vi"("Position"=w828, "Image In"=w833) -> ("RGB"=w837:cluster{"R":u32, "G":u32, "B":u32})  [unwired: 1 in, 2 out]
        n429 = Divide(x=w837, y=255) -> (x/y=w834:cluster{"R":dbl, "G":dbl, "B":dbl})
        n430 = Format Into String(format string="vp%04d%04d", error in=w825, w827, w826) -> (resulting string=w831:string, error out=w830:errorcluster)  [unwired: 1 in]
        n431 = call "RGB-HSV.vi"("RGB"=w834) -> ("YUV"=→"YUV_Calc":cluster{"Y":sgl, "U":sgl, "V":sgl})  [unwired: 13 in, 1 out]
        n432 = call "SRV_Write_Comm.vi"("error in (no error)"=w830, "Command Sent"=w831, "SRV In"=w822) -> ("error out"=w823:errorcluster, "SRV Out"=w820:refnum<k5>)  [unwired: 6 in, 1 out]
        n433 = Bundle By Name(cluster=w819, "SRV"=w820) -> (w821:T8)
      }
      frame #24 {
        n434 = call "SRV_Main Config Paths.vi"("local data"=w839) -> ("SystemConfig Filepath"=w838:path)  [unwired: 8 in, 6 out]
        n435 = call "SRV_System Config GUI.vi"("System Config File Path in"=w838) -> ("error out"=w844:errorcluster, "Cancelled?"=w840:bool)  [unwired: 8 in, 1 out]
        n436 = Select(t=w845, s=w845, f=w844) -> (s? t:f=w843:errorcluster)
        n437 = case "Cancelled?" shown="False" w840 {
          tunnel: w843 -> [w849 w850]
          tunnel: [w848 w850] -> w842
          tunnel: w841 -> [w847 _]
          frame #0 {
            n438 = call "SRV_Queue_Enqueue Element.vi"("error in (no error)"=w849, "Command"="InitTCP", "Command-Data Queue"=w847) -> ("error out"=w848:errorcluster)  [unwired: 6 in, 2 out]
          }
          frame #1 {
          }
        }
      }
      frame #25 {
        n439 = call "SRV_Main Config Paths.vi"("local data"=w852) -> ("MotorsConfig Filepath"=w851:path)  [unwired: 8 in, 6 out]
        n440 = call "SRV_Motors Config GUI.vi"("Motors Config File Path in"=w851) -> ("error out"=w857:errorcluster, "Cancelled?"=w853:bool)  [unwired: 8 in, 1 out]
        n441 = Select(t=w858, s=w858, f=w857) -> (s? t:f=w856:errorcluster)
        n442 = case "Cancelled?" shown="False" w853 {
          tunnel: w856 -> [w862 w863]
          tunnel: [w861 w863] -> w855
          tunnel: w854 -> [w860 _]
          frame #0 {
            n443 = call "SRV_Queue_Enqueue Element.vi"("error in (no error)"=w862, "Command"="InitMotors", "Command-Data Queue"=w860) -> ("error out"=w861:errorcluster)  [unwired: 6 in, 2 out]
          }
          frame #1 {
          }
        }
      }
      frame #26 {
        n444 = call "SRV_Main Config Paths.vi"("local data"=w865) -> ("SensorsConfig Filepath"=w864:path)  [unwired: 8 in, 6 out]
        n445 = call "SRV_Sensors Config GUI.vi"("Sensors Config File Path in"=w864) -> ("error out"=w870:errorcluster, "Cancelled?"=w866:bool)  [unwired: 8 in, 1 out]
        n446 = Select(t=w871, s=w871, f=w870) -> (s? t:f=w869:errorcluster)
        n447 = case "Cancelled?" shown="False" w866 {
          tunnel: w869 -> [w873 w879]
          tunnel: [w872 w879] -> w868
          tunnel: w867 -> [_ _]
          frame #0 {
            n448 = call "SRV_VIG_Sensor View Tab Open.vi"() -> ("Sensor View Tab Open?"=w874:bool)  [unwired: 14 in, 1 out]
            n449 = case "Sensor View Tab Open?" shown="True" w874 {
              tunnel: w873 -> [w875 w878]
              tunnel: [w875 w877] -> w872
              frame #0 {
              }
              frame #1 {
                n450 = call "SRV_SensorsQueue_Enqueue Element.vi"("error in (no error)"=w878, "Command"="Initialize") -> ("error out"=w877:errorcluster)  [unwired: 9 in]
              }
            }
          }
          frame #1 {
          }
        }
      }
      frame #27 {
        n451 = Unbundle By Name(w898) -> ("SRV"=w895:refnum<k5>, "true refs"=w891:refnum<vi>[], "Motor Control Config"=w884:T9[])
        n452 = Variant To Data(error in=w892, Variant=w893, type=T21 {"Button NewVal"=FALSE, "Button Index"=-1} ("Button Event Data")) -> (error out=w887:errorcluster, data=w888:T21)
        n453 = Unbundle By Name(w888) -> ("Button Index"=w885:i32, "Button NewVal"=w883:bool)
        n454 = Index Array(array=w891, index=w885) -> (element=w890:refnum<vi>)
        n455 = Index Array(array=w884, index=w885) -> (element=w881:T9)
        n456 = case shown="True" w883 {
          tunnel: w881 -> [w900 w902]
          tunnel: [w899 w901] -> w882
          frame #0 {
            n457 = Unbundle By Name(w900) -> ("Press Cmds.Motor Control Commands Array"=w899:T12[])
          }
          frame #1 {
            n458 = Unbundle By Name(w902) -> ("Release Cmds.Motor Control Commands Array"=w901:T12[])
          }
        }
        n459 = property class="Ring (strict)"(reference=w890, error in=w887, "Visible"=w883) -> (error out=w886:errorcluster)  [unwired: 1 out]
        n460 = Unbundle By Name(w881) -> ("Motor Type"=w880:T10)
        n461 = call "SRV_Execute Multiple Motor Control Commands.vi"("SRV"=w895, "Motor Type"=w880, "Motor Control Commands"=w882, "error in (no error)"=w886) -> ("SRV Out"=w896:refnum<k5>, "error out"=w894:errorcluster)  [unwired: 9 in, 1 out]
        n462 = Bundle By Name(cluster=w898, "SRV"=w896) -> (w897:T8)
      }
      frame #28 {
        n463 = call "SRV_SensorsQueue_Enqueue Element.vi"("Ignore Error 1? (F)"=TRUE, "error in (no error)"=w908, "Command"="Exit") -> ("error out"=w906:errorcluster)  [unwired: 8 in]
        n464 = flat-sequence {
          tunnel: w906 -> [w911]
          tunnel: [w911] -> w905
          frame #0 {
            n465 = call "SRV_Update Streaming States VIG.vi"("Enabled"=FALSE, "Streaming Modes"=SRV_Streaming_Modes."Sensors") -> ()  [unwired: 14 in]
          }
        }
        n466 = call "SRV_Wait (ms)+.vi"("milliseconds to wait"=u32 100, "error in (no error)"=w905) -> ("error out"=w904:errorcluster)  [unwired: 12 in, 1 out]
      }
      frame #29 {
        n467 = call "SRV_VIG_XModem Updates in Progress.vi"("XModem Updates in Progress"=TRUE, "Method (Get)"=enum16{"Get", "Set"}."Set") -> ()  [unwired: 12 in, 2 out]
        n468 = call "SRV_VIG_Streaming States.vi"() -> ("Streaming States out"=w916:T13)  [unwired: 15 in]
        n469 = Bundle By Name(cluster=w918, "Cached Streaming States"=w916) -> (w917:T8)
      }
      frame #30 {
        n470 = Unbundle By Name(w928) -> ("Cached Streaming States"=w927:T13)
        n471 = call "SRV_Queue Streaming Restore States.vi"("error in (no error)"=w925, "Cached Streaming States"=w927, "Control Queue"=w926) -> ("error out"=w923:errorcluster)  [unwired: 7 in, 1 out]
        n472 = call "SRV_VIG_XModem Updates in Progress.vi"("XModem Updates in Progress"=FALSE, "Method (Get)"=enum16{"Get", "Set"}."Set") -> ()  [unwired: 12 in, 2 out]
        n473 = property on="Show Image" class="Bool (strict)"(error in=w923, "DisabledEnum"=T17."Enabled" ("Disabled")) -> (error out=w922:errorcluster)  [unwired: 1 in, 1 out]
      }
      frame #31 {
        n474 = Format Into String(format string="Developer Error: The command \"%s\" is undefined for the SRV Control Queue.", w932) -> (resulting string=w930:string)  [unwired: 2 in, 1 out]
        n475 = call "SRV_Generate Error.vi"("Message"=w930, "error in (no error)"=w929) -> ("error out"=w931:errorcluster)  [unwired: 13 in]
      }
      frame #32 {
        n476 = Unbundle By Name(w935) -> ("SRV"=w938:refnum<k5>)
        n477 = call "SRV_Close TCP Connection.vi"("error in"=w940, "connection ID"=w938) -> ("error out"=w939:errorcluster)  [unwired: 9 in]
        n478 = Bundle By Name(cluster=w935, "SRV"=refnum<k5> refnum ("SRV Out")) -> (w937:T8)
      }
      frame #33 {
        n479 = Unbundle By Name(w956) -> ("button refs"=w943:refnum<vi>[], "false refs"=w942:refnum<vi>[], "true refs"=w941:refnum<vi>[], "Status"=w955:refnum<vi>)
        n480 = global read "SRVGlobals.vi" "Connected SRV IP"() -> (w966:string[])
        n481 = call "SRV_Update Status Indicator.vi"("Status ref"=w955, "Status"="Exiting...", "error in (no error)"=w964) -> ("error out"=w954:errorcluster)  [unwired: 11 in, 1 out]
        n482 = Release Queue(queue=w952, error in (no error)=w954) -> (error out=w953:errorcluster)  [unwired: 1 in, 2 out]
        n483 = for {
          tunnel: w966 -> [w977] mode=indexing
          shift-right: [w974] -> _
          shift-left: errorcluster {"status"=FALSE, "code"=0, "source"=""} ("error out") -> [w975]
          n484 = call "SRV_Reset TCP Connection.vi"("IP address"=w977) -> ("error out"=w976:errorcluster)  [unwired: 9 in, 1 out]
          n485 = Select(t=w975, s=w975, f=w976) -> (s? t:f=w974:errorcluster)
        }
        n486 = Release Queue(queue=w957, error in (no error)=w953) -> (error out=w958:errorcluster)  [unwired: 1 in, 2 out]
        n487 = call "SRV_Number of IMJ Requests Methods.vi"("Number of IMJ Requests ref"=w959, "semaphore ref"=w960, "error in (no error)"=w958, "Number of IMJ Requests Methods (Read)"=SRV_Number_of_IMJ_Requests_Methods."Close") -> ("error out"=w945:errorcluster)  [unwired: 7 in, 4 out]
        n488 = disable-structure shown="Disabled" {
          disable-tunnel: w945 -> [w972 w973]
          disable-tunnel: [w971 w973] -> w944
          disable-tunnel: w943 -> [w970 _]
          disable-tunnel: w942 -> [w969 _]
          disable-tunnel: w941 -> [w968 _]
          frame #0 {
            n489 = call "SRV_Shutdown Motor Buttons.vi"("button refs"=w970, "false refs"=w969, "true refs"=w968, "error in (no error)"=w972) -> ("error out"=w971:errorcluster)  [unwired: 11 in]
          }
          frame #1 {
          }
        }
        n490 = call "SRV_SRV_Loops Notifier.vi"("Notifier Methods"=SRV_SRV_Loops_Notifier_Methods."Release Notifier", "error in (no error)"=w944) -> ("error out"=w951:errorcluster)  [unwired: 8 in, 1 out]
        n491 = call "SRV_SRV_zZ Notifier.vi"("Notifier Methods"=SRV_SRV_Loops_Notifier_Methods."Release Notifier", "error in (no error)"=w951) -> ("error out"=w949:errorcluster)  [unwired: 9 in]
        n492 = call "SRV_SensorsQueue_Enqueue Element.vi"("Ignore Error 1? (F)"=TRUE, "error in (no error)"=w949, "Command"="Exit") -> ("error out"=w948:errorcluster)  [unwired: 8 in]
      }
    }
    n493 = Unbundle By Name(w350) -> ("SRV"=w349:refnum<k5>)
    n494 = Not A Number/Path/Refnum?(number/path/refnum=w349) -> (NaN/Path/Refnum?=w364:bool)
    n495 = Not(x=w364) -> (.not. x?=→"connected?":bool)
    n496 = call "SRV_Manage Loop Errors.vi"("Loop Identifier"="Control Loop", "error in (no error)"=w346) -> ("error out"=w352:errorcluster)  [unwired: 9 in]
    "i2" <- w357
  }
  n497 = while {
    shift-right: [w1014] -> _
    shift-left: w110 -> [w1015]
    tunnel: w109 -> [w1012]
    tunnel: [w1009] -> w115
    tunnel: w141 -> [w1007]
    shift-right: [w1000] -> _
    shift-left: w111 -> [w990]
    tunnel: w124 -> [w1004]
    tunnel: w142 -> [w1003]
    tunnel: w139 -> [w997]
    tunnel: w114 -> [w991]
    i -> [w1008]
    stop <- w1013 stop-if-true
    # "# IMJ Requests sema"
    # "# IMJ Requests ref"
    # "SRV IP"
    n498 = call "SRV_ms Timer.vi"("error in (no error)"=w990) -> ("ms Tick"=w984:u32, "error out"=w989:errorcluster)  [unwired: 16 in, 1 out]
    n499 = call "SRV_PM_Dequeue and Parse Packet.vi"("SRV_Packets queue"=w991, "error in (no error)"=w989) -> ("Packet"=w999:T16, "Data String"=w998:string, "error out"=w986:errorcluster)  [unwired: 4 in, 7 out]
    n500 = case shown="\"New PM\"" w997 {
      tunnel: w1012 -> [w1020 w1021]
      tunnel: [w1019 w1021] -> w1011
      frame #0 {
        n501 = call <vilib>:"Acquire Semaphore.vi"("semaphore"=w1020) -> ("semaphore out"=w1019:T20)  [unwired: 4 in, 2 out]
      }
      frame #1 {
        # "TCP Read sema"
      }
    }
    n502 = call "SRV_PM_VIG_WIP Byte Array Size.vi"() -> ("WIP Size out"=w980:i32)  [unwired: 10 in, 1 out]
    n503 = call "SRV_ms Timer.vi"("ms Previous Tick"=w984, "error in (no error)"=w986) -> ("ms Tick"=w983:u32, "ms Diff"=→"ms Diff DQ":u32, "error out"=w985:errorcluster)  [unwired: 15 in]
    n504 = call "SRV_Determine Incoming Data Type.vi"("Data"=w998, "error in (no error)"=w985) -> ("Data dup"=w996:string, "Response Data Type"=w993:T3, "error out"=w994:errorcluster)  [unwired: 11 in]
    n505 = Greater?(x=w980, y=100000) -> (0:→"Overflow Indicator":bool)
    n506 = call "SRV_Send No Data if Shutdown.vi"("Data"=w996, "Response Data Type"=w993, "error in (no error)"=w994) -> ("Data dup"=w995:string, "Response Data Type out"=w992:T3, "error out"=w988:errorcluster)  [unwired: 10 in]
    "Response Data Type" <- w992
    n507 = call "SRV_ms Timer.vi"("ms Previous Tick"=w983, "error in (no error)"=w988) -> ("ms Diff"=→"ms Diff parse":u32, "error out"=w987:errorcluster)  [unwired: 15 in, 1 out]
    n508 = case shown="\"#NA\"..\"##R,\"" w992 {
      selector: w992 -> [_ _ _ _ _ _ w1101 _]
      tunnel: w1015 -> [w1029 w1039 w1074 w1081 w1093 w1099 w1106 w1124]
      tunnel: [w1023 _ w1068 w1078 w1084 w1095 _ w1122] -> w1006
      tunnel: [_ _ _ _ _ _ _ w1113] -> w1013
      tunnel: [w1029 w1039 w1074 w1081 w1093 w1099 w1106 w1124] -> w1014
      tunnel: w1011 -> [w1028 w1040 w1073 w1080 w1092 w1098 w1105 w1123]
      tunnel: [w1028 w1040 w1073 w1080 w1092 w1098 w1105 w1123] -> w1010
      tunnel: w1007 -> [_ w1037 _ _ _ _ _ _]
      tunnel: [w1026 w1032 w1072 w1079 w1082 w1096 w1103 w1114] -> w1005
      tunnel: w987 -> [w1027 w1035 w1072 w1079 w1083 w1097 w1104 w1115]
      tunnel: w1003 -> [_ w1036 _ _ _ _ _ _]
      tunnel: w999 -> [_ _ _ _ _ _ _ _]
      tunnel: w995 -> [w1024 w1038 w1069 w1078 w1084 w1095 w1102 w1122]
      frame #0 {
        n509 = call "SRV_Shutdown Flag.vi"("error in (no error)"=w1027) -> ("Shutdown Flag out"=w1025:bool, "error out"=w1026:errorcluster)  [unwired: 13 in]
        n510 = Select(t="", s=w1025, f=w1024) -> (s? t:f=w1023:string)
      }
      frame #1 {
        n511 = call "SRV_ms Timer.vi"("error in (no error)"=w1035) -> ("ms Tick"=w1031:u32, "error out"=w1034:errorcluster)  [unwired: 16 in, 1 out]
        n512 = flat-sequence {
          tunnel: w1039 -> [w1058]
          tunnel: w1034 -> [w1051]
          tunnel: [w1041] -> w1033
          tunnel: w1038 -> [w1056]
          tunnel: w1037 -> [_]
          tunnel: w1036 -> [_]
          frame #0 {
            # "TCP Reads if using old non-packet mode"
            # "grab JPEG compressed video frame"
            n513 = call "SRV_ms Timer.vi"("error in (no error)"=w1051) -> ("ms Tick"=w1047:u32, "error out"=w1050:errorcluster)  [unwired: 16 in, 1 out]
            n514 = call "SRV_Get TCP Connection.vi"("error in (no error)"=w1050, "IP address"=w1058) -> ("error out"=w1049:errorcluster, "connection ID"=w1057:refnum<k5>)  [unwired: 8 in]
            n515 = call "SRV_ms Timer.vi"("ms Previous Tick"=w1047, "error in (no error)"=w1049) -> ("ms Tick"=w1055:u32, "ms Diff"=→"ms Diff 2":u32, "error out"=w1052:errorcluster)  [unwired: 15 in]
            n516 = call "SRV_Get and Show Image.vi"("Connection ID"=w1057, "Data"=w1056, "error in (no error)"=w1052) -> ("Image/Movie Out"=w1060:T7, "image"=w1059:picture, "dimensions"=w1061:cluster{"Witdh":i32, "Height":i32}, "error out"=w1053:errorcluster)  [unwired: 8 in, 1 out]
            n517 = call "SRV_ms Timer.vi"("ms Previous Tick"=w1055, "error in (no error)"=w1053) -> ("ms Tick"=w1048:u32, "ms Diff"=→"ms Diff":u32, "error out"=w1045:errorcluster)  [unwired: 15 in]
            n518 = flat-sequence {
              tunnel: w1061 -> [w1067]
              tunnel: w1060 -> [w1066]
              tunnel: w1059 -> [w1065]
              tunnel: [w1062] -> w1042
              tunnel: w1048 -> [w1063]
              tunnel: w1045 -> [w1064]
              tunnel: [w1063] -> w1044
              frame #0 {
                n519 = property on="The image" class="Picture"("Draw Area Size"=w1067) -> ()  [unwired: 2 in, 2 out]
                n520 = call <vilib>:"Clear Errors.vi"("error in (no error)"=w1064) -> ("error out"=w1062:errorcluster)  [unwired: 6 in]
                "Image/Movie Out" <- w1066
                "The image" <- w1065
              }
            }
            n521 = call "SRV_ms Timer.vi"("ms Previous Tick"=w1044, "error in (no error)"=w1042) -> ("ms Diff"=→"ms Diff 3":u32, "error out"=w1041:errorcluster)  [unwired: 15 in, 1 out]
          }
        }
        n522 = call "SRV_ms Timer.vi"("ms Previous Tick"=w1031, "error in (no error)"=w1033) -> ("ms Diff"=→"ms Diff ##IMJ":u32, "error out"=w1032:errorcluster)  [unwired: 15 in, 1 out]
      }
      frame #2 {
        # "Read the contents of the PicoC printf() buffer and clear it.\n\nThis command causes the contents of the PicoC buffered serial stream (from printf() and output() calls in PicoC, when the buffered mode is enabled) to be send in the reply. Note that the reply can be up to 64KB long. After the entire contents of the buffer are sent in the reply, the buffer is cleared.\n\n[length] is an ASCII value from 0 to 65525 and it indicates the number of bytes in [buffer_data].\n\n[buffer_data] is the entire contents of the serial stream buffer, and can include any data bytes"
        n523 = call "SRV_Parse Response (B).vi"("#B Data in"=w1069) -> ("number of bytes in buffer_data"=w1071:i32, "Beginning of buffer_data"=w1070:string)  [unwired: 4 in, 5 out]
        n524 = case shown="..0" w1071 {
          tunnel: w1070 -> [_ w1076]
          tunnel: ["" w1076] -> w1068
          frame #0 {
          }
          frame #1 {
          }
        }
      }
      frame #3 {
        # "Execute C Program\n\nRuns the PicoC program stored in flash buffer, which got there via the 'E' line editor, the 'zr' or 'zRxx' command (which reads a flash sector into flash buffer) or 'X' command (XMODEM file transfer). PicoC program must have an exit(1); call to return control to the main firmware.\n\nWhen PicoC Background Mode mode is active (simultainous PicoC and Firmware commands), you must send a '|' character to get PicoC to exit before the exit(); call in the code. When PicoC Background Mode is not active (only PicoC running, Firmware commands ignored), you have to send an 'ESC' to terminate the PicoC program before the exit(); call runs.\n\nWhen PicoC exits, the SRV will send the string \"##Leaving PicoC\\r\\n\", which indicates to the client that the PicoC program exited normally.\n \n'|'  Break out of running PicoC program\n\nIf a PicoC program is running and PicoC Background Mode is active, you can send the '|' character to the firmware and at the next statement, the PicoC program will exit and return \"##Leaving PicoC\\r\\n\"."
        n525 = local write "In Pico"(FALSE ("Enable?")) -> ()
      }
      frame #4 {
        # "RGB\n\n##vp yyy uuu vvv\\r\\n\n\nthe 'vp' command samples a single pixel defined by coordinates xxxx (column 0000-0159, 0000-0319, 0000-0639, 0000-1279 depending on resolution) and yy (row 0000-0127, 0000-0255, 0000-0511, 0000-1023, where 0000 is top of image). 'vp01600128' will sample a pixel in the middle of the image at 320x256 resolution, 'vp01600000' will sample a pixel in the middle of the top row, etc..."
        n526 = Match Pattern(string=w1084, regular expression="vp " ("Command Sent")) -> (after substring=w1085:string)  [unwired: 1 in, 3 out]
        n527 = Scan From String(input string=w1085, error in=w1083) -> (error out=w1091:errorcluster, output 1=w1089:dbl, output 2=w1088:dbl, output 3=w1087:dbl)  [unwired: 5 in, 2 out]
        n528 = Bundle(w1089, w1088, w1087) -> (→"YUV_SRV":cluster{dbl, dbl, dbl})  [unwired: 1 in]
        n529 = call <vilib>:"Clear Errors.vi"("error in (no error)"=w1091) -> ("error out"=w1082:errorcluster)  [unwired: 6 in]
      }
      frame #5 {
        # "##zZ\\r\\n\n\nflash memory boot sector update - writes contents of flash buffer to boot sectors of flash memory - used to replace u-boot.ldr or srv1.ldr - checks first that a valid LDR format image is in the flash buffer"
        n530 = call "SRV_SRV_zZ Notifier.vi"("Notifier Methods"=SRV_SRV_Loops_Notifier_Methods."Send Notification", "error in (no error)"=w1097, "Notification String"=w1095) -> ("error out"=w1096:errorcluster)  [unwired: 8 in]
      }
      frame #6 {
        # "#NA\n##$A\n#Nb\n##iL\n##iL\n##NP,\n##R,"
        n531 = call "SRV_VIG_Sensor View Tab Open.vi"() -> ("Sensor View Tab Open?"=w1100:bool)  [unwired: 14 in, 1 out]
        n532 = case "Sensor View Tab Open?" shown="True" w1100 {
          tunnel: w1104 -> [w1107 w1112]
          tunnel: [w1107 w1111] -> w1103
          tunnel: w1102 -> [_ w1110]
          tunnel: w1101 -> [_ w1108]
          frame #0 {
          }
          frame #1 {
            n533 = Format Into String(w1108) -> (resulting string=w1109:string)  [unwired: 3 in, 1 out]
            n534 = call "SRV_SensorsQueue_Enqueue Element.vi"("error in (no error)"=w1112, "Data"=w1110, "Command"=w1109) -> ("error out"=w1111:errorcluster)  [unwired: 8 in]
          }
        }
      }
      frame #7 {
        n535 = Unbundle By Name(w1115) -> ("status"=w1119:bool, "code"=w1121:i32)
        n536 = call "SRV_Shutdown Flag.vi"("error in (no error)"=w1115) -> ("Shutdown Flag out"=w1113:bool, "error out"=w1116:errorcluster)  [unwired: 13 in]
        n537 = Equal?(x=w1121, y=1122 ("code (42: generic error)")) -> (x = y?=w1118:bool)
        n538 = Compound Arithmetic op=AND(w1119, w1118, w1113) -> (w1117:bool)
        n539 = case shown="True" w1117 {
          tunnel: w1116 -> [w1125 w1127]
          tunnel: [w1125 w1126] -> w1114
          frame #0 {
          }
          frame #1 {
            # "Shutting Down"
            n540 = call <vilib>:"Clear Errors.vi"("error in (no error)"=w1127) -> ("error out"=w1126:errorcluster)  [unwired: 6 in]
          }
        }
      }
    }
    n541 = call "SRV_Update Replies Indicator.vi"("Replies ref"=w1004, "Text to Append"=w1006, "error in (no error)"=w1005) -> ("error out"=w1001:errorcluster)  [unwired: 11 in, 1 out]
    n542 = case shown="\"New PM\"" w997 {
      tunnel: w1010 -> [w1017 w1018]
      tunnel: [w1016 w1018] -> w1009
      frame #0 {
        n543 = call <vilib>:"Release Semaphore.vi"("semaphore"=w1017) -> ("semaphore out"=w1016:T20)  [unwired: 5 in, 1 out]
      }
      frame #1 {
      }
    }
    n544 = call "SRV_Manage Loop Errors.vi"("Loop Identifier"="Receive Action Loop", "error in (no error)"=w1001) -> ("error out"=w1000:errorcluster)  [unwired: 9 in]
    "i4" <- w1008
  }
  n545 = Unregister For Events(event registration refnum=w129, error in=w130) -> ()  [unwired: 1 out]
  n546 = Unbundle By Name(w127) -> ("Main Controller ref"=w112:refnum<vi>, "user event"=w126:refnum<user-event>)
  n547 = flat-sequence {
    tunnel: w140 -> [_]
    tunnel: w128 -> [_]
    tunnel: w126 -> [w1134]
    tunnel: [w1129] -> w125
    tunnel: w115 -> [w1128]
    tunnel: w107 -> [_]
    tunnel: w125 -> [_]
    tunnel: w112 -> [w1136]
    frame #0 {
      n548 = call "SRV_Generate User Exit Event.vi"("User Exit Event"=w1134) -> ("error out"=w1132:errorcluster, "User Exit Event out"=w1130:refnum<user-event>)  [unwired: 9 in]
      n549 = call "SRV_Wait (ms)+.vi"("milliseconds to wait"=u32 100 ("Delay (ms)"), "error in (no error)"=w1132) -> ("error out"=w1131:errorcluster)  [unwired: 12 in, 1 out]
      n550 = call <vilib>:"Release Semaphore Reference.vi"("semaphore"=w1128) -> ()  [unwired: 9 in, 2 out]
      n551 = Destroy User Event(user event=w1130, error in=w1131) -> (error out=w1129:errorcluster)
      "Status" <- ""
    }
    frame #1 {
      w1137 = FALSE  # Close When Done?
      # "Don't Close is the behavior desired by T Jump (Feb2014)"
      n552 = case shown="True" w1137 {
        tunnel: w1136 -> [_ w1138]
        frame #0 {
        }
        frame #1 {
          n553 = invoke class="VI" method="FP.Close"(reference=w1138) -> ()  [unwired: 2 in, 3 out]
        }
      }
    }
  }
